vi "OdorSystem-V2.2.vi"() -> ()   [LabVIEW 2019]
doc: "Control odor delivery system in Setup B\n\nNeeds Labview 2019 and DAQmx 19! So that it is compatible with scanimage on Setup B\n\nBy Dr. Jan Eckhardt, Group Friedrich, FMI Basel"
uses:
  StatesEnum.ctl
  <vilib>/vision/Avi.llb/IMAQ AVI2 Refnum.ctl
  <vilib>/Utility/error.llb/DialogType.ctl
  <vilib>/DAQmx/write.llb/DAQmx Write (Digital 1D Bool NChan 1Samp 1Line).vi
  <vilib>/DAQmx/write.llb/DAQmx Write (Digital Wfm 1Chan NSamp).vi
  <vilib>/DAQmx/read.llb/DAQmx Read (Counter U32 1Chan 1Samp).vi
  <vilib>/DAQmx/read.llb/DAQmx Read (Digital 1D Bool 1Chan 1Samp).vi
  <vilib>/Utility/config.llb/Read Key (Double).vi
  <vilib>/Utility/config.llb/Read Key (I32).vi
  <vilib>/Utility/config.llb/Read Key (Boolean).vi
  <vilib>/Utility/config.llb/Read Key (String).vi
  <vilib>/DAQmx/miscellaneous.llb/DAQmx Fill In Error Info.vi
  <vilib>/DAQmx/create/channels.llb/DAQmx Create Channel (CO-Pulse Generation-Frequency).vi
  <vilib>/Waveform/DWDTOps.llb/Digital Pattern Generator (Single Value).vi
  <vilib>/Waveform/DWDTOps.llb/DWDT Append Digital Samples.vi
  <vilib>/DAQmx/configure/timing.llb/DAQmx Timing (Implicit).vi
  <vilib>/DAQmx/create/channels.llb/DAQmx Create Channel (CI-Count Edges).vi
  <vilib>/DAQmx/configure/timing.llb/DAQmx Timing (Sample Clock).vi
  <vilib>/Waveform/DWDTOps.llb/DWDT Append Digital Signals.vi
  <vilib>/Waveform/DWDTOps.llb/DWDT Digital to Boolean Array.vi
  <vilib>/DAQmx/create/channels.llb/DAQmx Create Channel (DO-Digital Output).vi
  <vilib>/Waveform/DWDTOps.llb/DWDT Uncompress Digital.vi
  <resource>/objmgr/daqmx.rc
  <vilib>/Utility/config.llb/NI_LVConfig.lvlib
  <vilib>/vision/driver/NI_Vision_Acquisition_Software.lvlib
panel:
  in  "Save Video as":enum32{"Bin", "Avi"}(radio)
  out "Experiment Refnum":T1
  in  "Start Recording":bool
  in  "Avi Codec":u16(ring)=3 items=["Intel IYUV codec", "Microsoft Video 1", "FF Video Codec 1 (FFV1) (NI Vision)", "Motion JPEG (NI Vision)", "VP8 (NI Vision)", "VP9 (NI Vision)", "Y800 Uncompressed Grey Scale (NI Vision)", "YUV 4:2:0 Planar (NI Vision)"]
  in  "Basename":string="Test5_Fish2_comparison"
  in  "Video path":path=path "C:/Users/eckhjan/Setup-C/output/JanVersion"
  in  "Image Type":T2 items=["Grayscale (U8)", "Grayscale (I16)", "Grayscale (SGL)", "Complex (CSG)", "RGB (U32)", "HSL (U32)", "RGB (U64)", "Grayscale (U16)"]
  out "Image":T3(plugin-control)
  in  "Time between frames (ms)":dbl(slide)=19.0 step=1.0 scale=0.0..100.0
  in  "Camera Name":refnum<k21> caption="IMAQdx Session"
  out "Loaded experiment":string
  in  "Load exp. ini":bool
  in  "Use Default valve":bool=TRUE
  in  "Selected default valve":u8(knob)=8 min=1 max=8 step=1 scale=1.0..8.0
  out "Framecount":u32
  in  "Image count filepath":path
  out "Experiment running":bool
  out "State":T4
  in  "Select experiment":enum32{"Single trial", "Trial series"}(tab)
  out "Time elapsed":dbl format="%.1f"
  in  "Start single trial":bool
  out "single trial done":bool
  in  "Select valve":u8(knob)=1 min=1 max=8 step=1 scale=1.0..8.0
  out "Pause elapsed time":dbl format="%#.1f"
  out "In between trials":bool
  out "Trial elapsed time":dbl format="%.1f"
  out "Total elapsed time":dbl format="%.1f"
  out "Estimated total time":dbl
  out "Current list index":i32
  out "Current Valve":u8
  in  "Time between trials":u16=10 min=1 max=900 step=1
  in  "Start trial series":bool
  in  "Valve order list":i8[](array[numeric]) min=1 max=8 step=1
  out "Digitaler output":digitalwaveform(graph)
  out "Stop Boolesch":bool
  in  "Total trial time":dbl=20.0 min=1.0 step=0.1
  in  "Valve opening time":dbl=10.0 min=0.0 step=0.1
  in  "Valve delay":dbl=2.0 min=0.0 step=0.1
  in  "Stopp":bool
  # "All times are in second!"
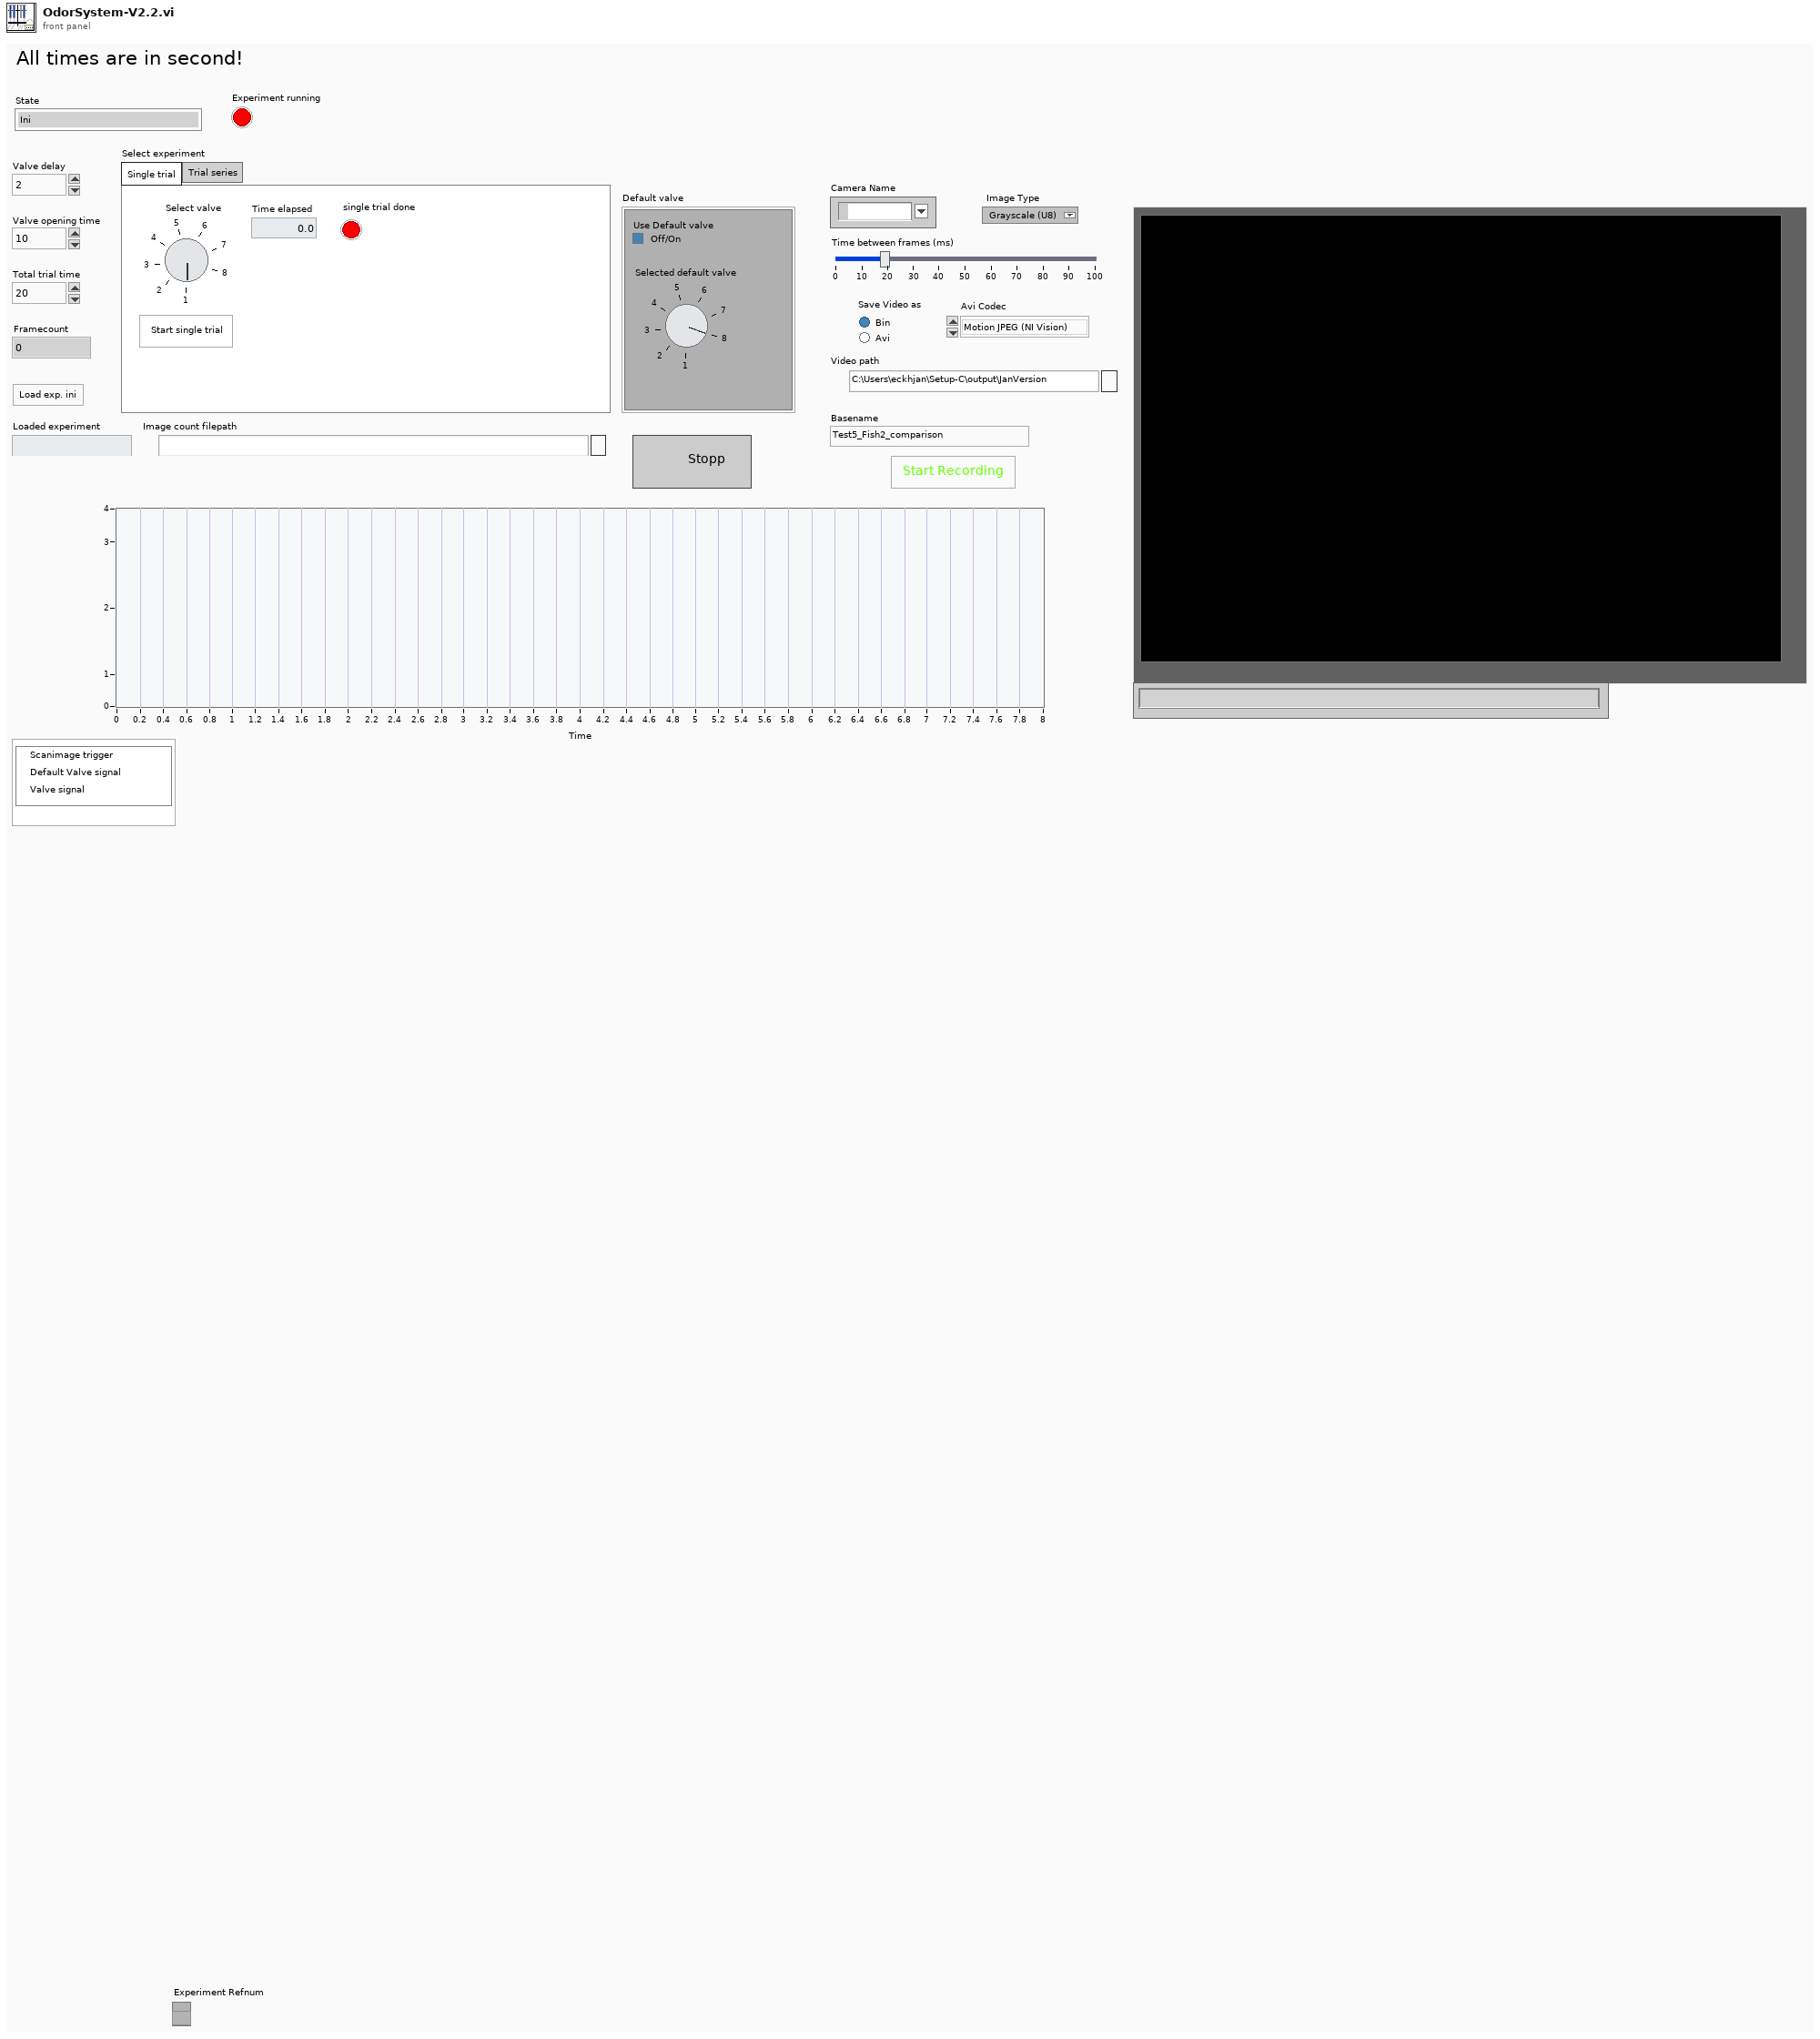
[diagram p1: front panel]
types:
  T1 = typedef "IMAQ AVI2 Refnum.ctl" = refnum<k20>
  T2 = typedef "Image Type" = u32
  T3 = typedef "IMAQ Image.ctl" = refnum<image>
  T4 = typedef "StatesEnum.ctl" = enum16{"Ini", "Standby", "Start Trial", "Start trial series", "Stop"}
  T5 = typedef "IMAQdx.ctl" = refnum<k21>
  T6 = enum8{"Enabled", "Disabled", "Disabled and Grayed Out"}
  T7 = enum32{"Page Enabled", "Page Disabled", "Page Disabled & Grayed"}
  T8 = enum16{"open", "replace", "create", "open or create", "replace or create", "replace or create with confirmation"}
  T9 = enum16{"big-endian, network order", "native, host order", "little-endian"}
  T10 = typedef "NI_LVConfig.lvlib/Config Data RefNum.ctl" = refnum<k1>
  T11 = typedef "DialogType.ctl" = u16
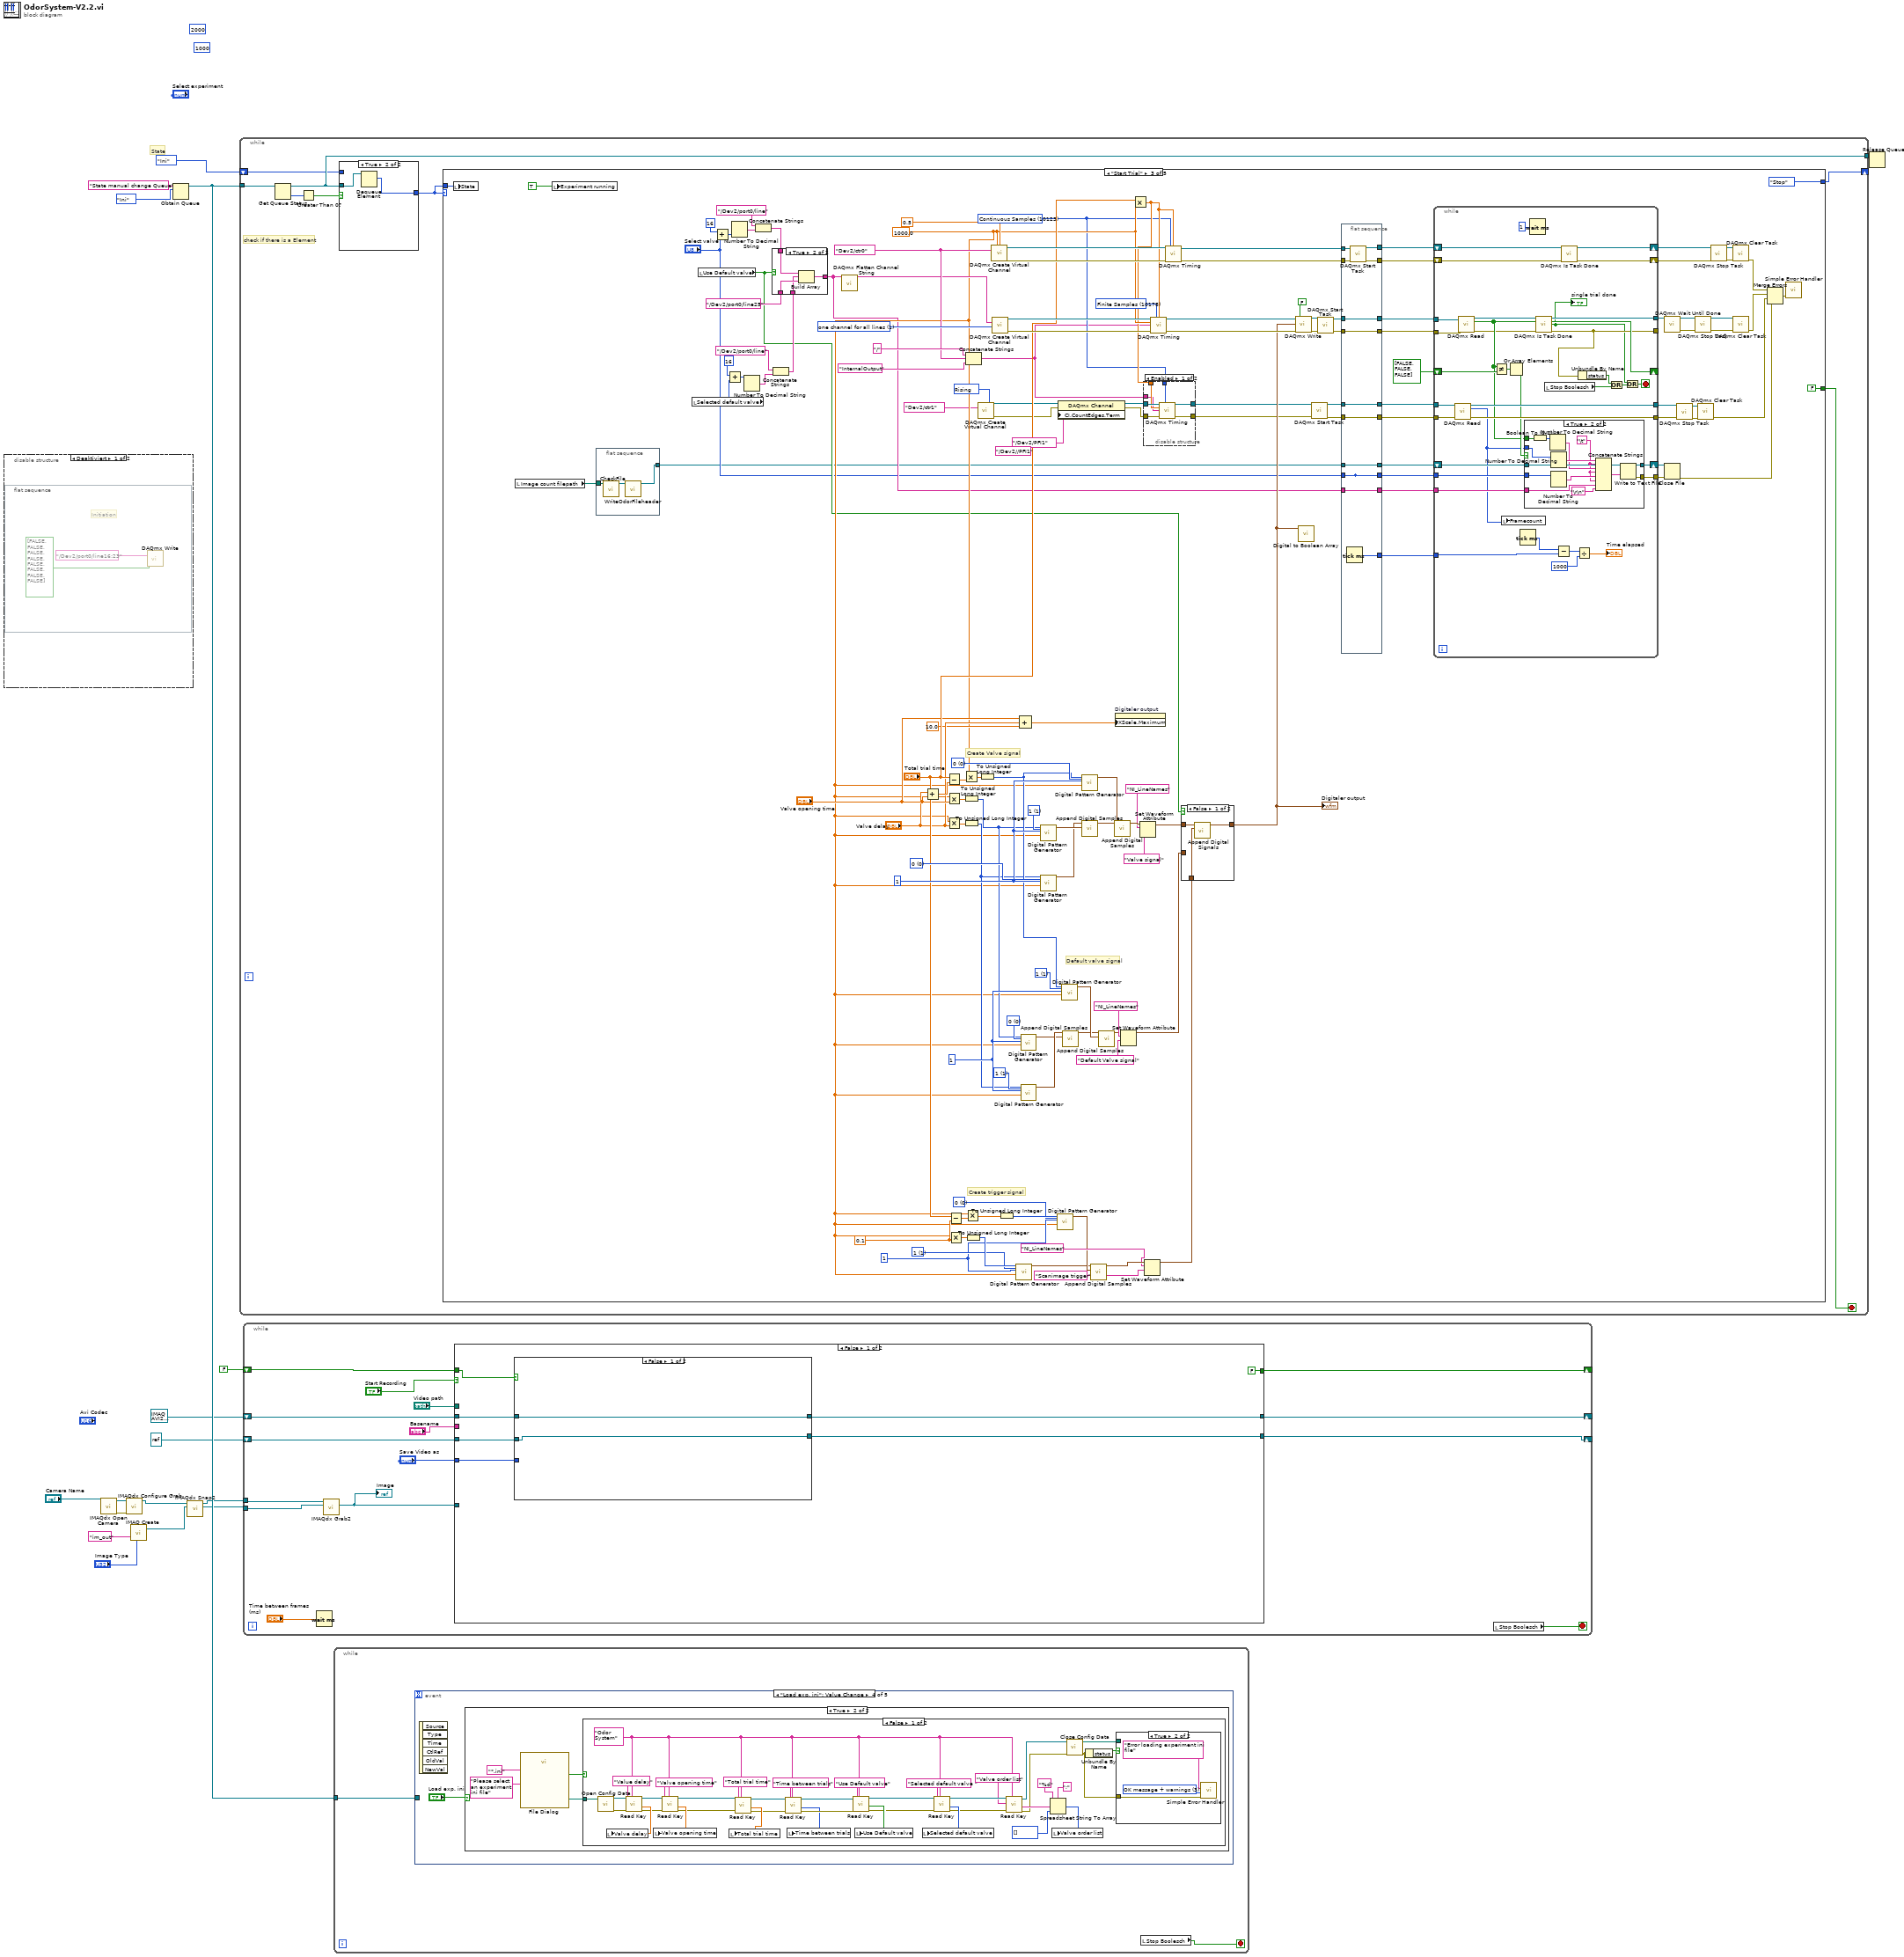
[diagram p0: block diagram]
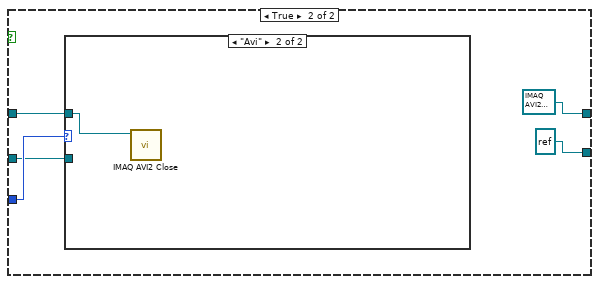
[diagram p2: hidden frame]
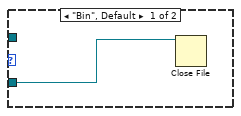
[diagram p3: hidden frame]
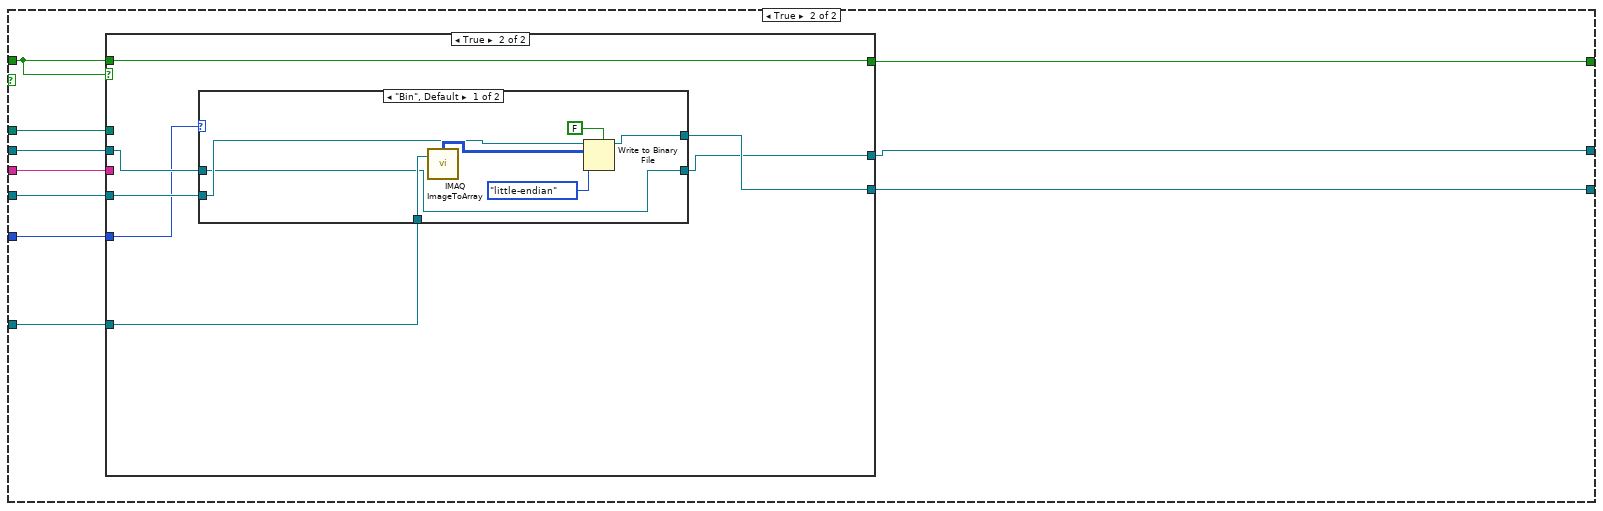
[diagram p4: hidden frame]
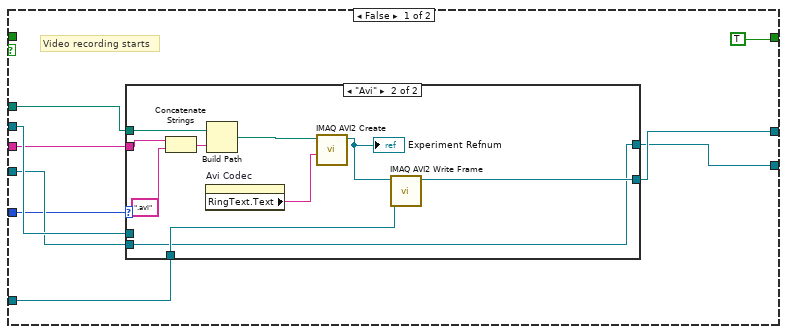
[diagram p5: hidden frame]
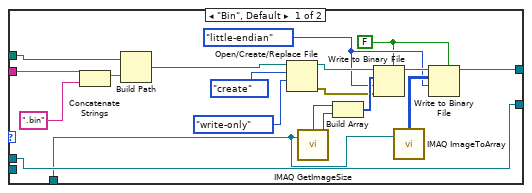
[diagram p6: hidden frame]
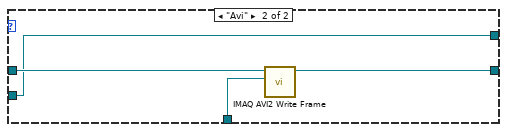
[diagram p7: hidden frame]
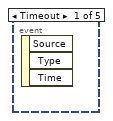
[diagram p9: hidden frame]
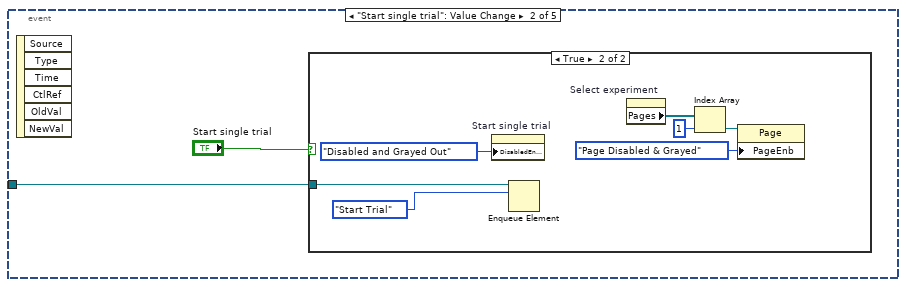
[diagram p10: hidden frame]
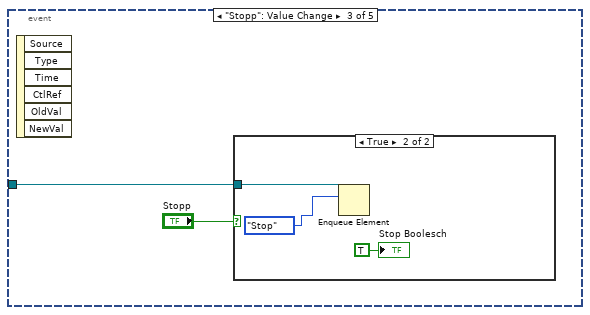
[diagram p12: hidden frame]
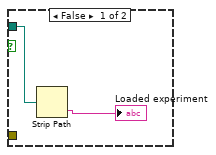
[diagram p15: hidden frame]
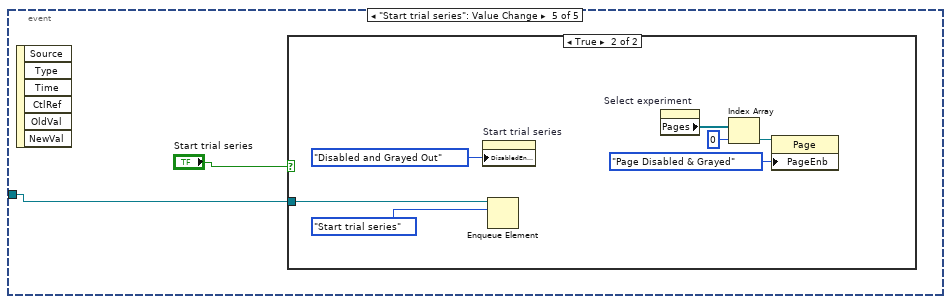
[diagram p17: hidden frame]
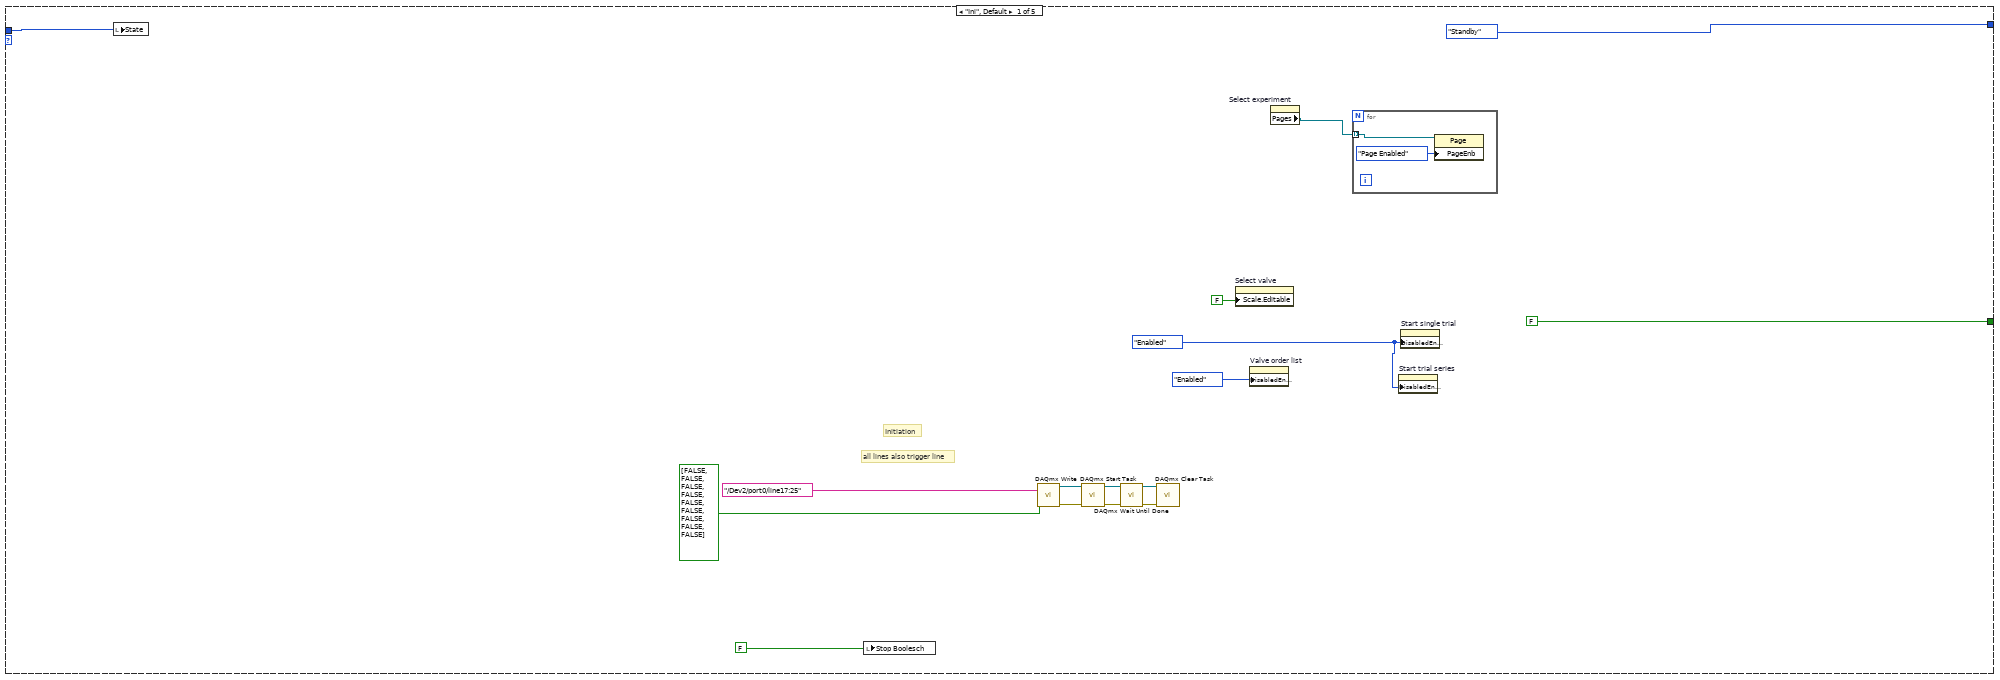
[diagram p20: hidden frame]
diagram:
  (unwired) u32 2000 ("number of samples")
  (unwired) u32 1000 ("number of samples")
  # "State"
  n1 = disable-structure shown="Deaktiviert" {
    frame Disabled {
      n2 = flat-sequence {
        frame #0 {
          # "Initiation"
          n3 = call-poly <vilib>:"DAQmx Write.vi"("task/channels in"="/Dev2/port0/line16:23" ("string"), "data"=bool[] [FALSE, FALSE, FALSE, FALSE, FALSE, FALSE, FALSE, FALSE]) -> ()  [unwired: 11 in, 3 out]
        }
      }
    }
    frame Enabled {
    }
  }
  n4 = call <vilib>:"IMAQdx Open Camera.vi"("Session In"="Camera Name") -> ("error out"=w11:errorcluster, "Session Out"=w12:T5)  [unwired: 9 in]
  n5 = call <vilib>:"IMAQdx Configure Grab.vi"("error in"=w11, "Session In"=w12) -> ("Session Out"=w5:T5)  [unwired: 8 in, 1 out]
  n6 = call "IMAQ Create"("Image Name"="im_out", "Image Type"="Image Type") -> ("New Image"=w4:T3)  [unwired: 3 in, 1 out]
  n7 = Obtain Queue(name (unnamed)="State manual change Queue", element data type=StatesEnum."Ini" ("Enum")) -> (queue out=w16:refnum<queue>)  [unwired: 3 in, 2 out]
  n8 = call <vilib>:"IMAQdx Snap2.vi"("Image In"=w4, "Session In"=w5) -> ("Image Out"=w2:T3, "Session Out"=w3:T5)  [unwired: 7 in, 1 out]
  n9 = while {
    tunnel: w16 -> [w25]
    tunnel: [w24] -> w15
    shift-right: [w20] -> _
    shift-left: StatesEnum."Ini" -> [w21]
    stop <- w23 stop-if-true
    # "check if there is a Element"
    n10 = Get Queue Status(queue=w25) -> (queue out=w24:refnum<queue>, # elements in queue=w27:i32)  [unwired: 2 in, 6 out]
    n11 = Greater Than 0?(x=w27) -> (x > 0?=w26:bool)
    n12 = case shown="True" w26 {
      tunnel: w24 -> [_ w30]
      tunnel: w21 -> [w28 _]
      tunnel: [w28 w29] -> w22
      frame False {
      }
      frame True {
        n13 = Dequeue Element(queue=w30) -> (element=w29:T4)  [unwired: 2 in, 3 out]
      }
    }
    n14 = case shown="\"Start Trial\"" w22 {
      tunnel: w22 -> [w41 w49 w127 w288 w607]
      tunnel: [FALSE ("Stop Boolesch") FALSE ("Stop Boolesch") FALSE ("Stop Boolesch") FALSE ("Stop Boolesch") w609] -> w23
      tunnel: [StatesEnum."Standby" ("Enum") w49 StatesEnum."Stop" ("Enum") StatesEnum."Stop" ("Enum") StatesEnum."Standby" ("Enum")] -> w20
      frame "Ini", Default {
        w34 = T6."Enabled" ("Deaktiviert")
        # "all lines also trigger line"
        # "Initiation"
        n15 = local write "State"(w41) -> ()
        n16 = local write "Stop Boolesch"(FALSE ("Stop Boolesch")) -> ()
        n17 = call-poly <vilib>:"DAQmx Write.vi"("task/channels in"="/Dev2/port0/line17:25" ("string"), "data"=bool[] [FALSE, FALSE, FALSE, FALSE, FALSE, FALSE, FALSE, FALSE, FALSE]) -> ("task out"=w36:refnum<k21>, "error out"=w35:errorcluster)  [unwired: 11 in, 1 out]
        n18 = call <vilib>:"DAQmx Start Task.vi"("task/channels in"=w36, "error in"=w35) -> ("task out"=w40:refnum<k21>, "error out"=w38:errorcluster)  [unwired: 12 in]
        n19 = call <vilib>:"DAQmx Wait Until Done.vi"("task/channels in"=w40, "error in"=w38) -> ("task out"=w39:refnum<k21>, "error out"=w37:errorcluster)  [unwired: 12 in]
        n20 = call <vilib>:"DAQmx Clear Task.vi"("task in"=w39, "error in"=w37) -> ()  [unwired: 13 in, 1 out]
        n21 = property on="Select valve" class="Knob (strict)"("Scale.Editable"=FALSE ("Skala.Editierbar")) -> ()  [unwired: 2 in, 2 out]
        n22 = property on="Valve order list" class="Arr (strict)"("DisabledEnum"=T6."Enabled" ("Deaktiviert")) -> ()  [unwired: 2 in, 2 out]
        n23 = property on="Select experiment" class="TabCtl (strict)"() -> ("Pages"=w32:refnum<vi>[])  [unwired: 2 in, 2 out]
        n24 = for {
          tunnel: w32 -> [w47] mode=indexing
          n25 = property class="Page"(reference=w47, "PageEnb"=T7."Page Enabled" ("Aktiv-Status der Seite")) -> ()  [unwired: 1 in, 2 out]
        }
        n26 = property on="Start trial series" class="Bool"("DisabledEnum"=w34) -> ()  [unwired: 2 in, 2 out]
        n27 = property on="Start single trial" class="Bool"("DisabledEnum"=w34) -> ()  [unwired: 2 in, 2 out]
      }
      frame "Standby" {
        n28 = local write "State"(w49) -> ()
        n29 = Wait (ms)(milliseconds to wait=u32 1 ("Zu wartende ms")) -> ()  [unwired: 1 out]
      }
      frame "Start Trial" {
        w95 = 10178 items=["Finite Samples"=10178, "Continuous Samples"=10123, "Hardware Timed Single Point"=12522] ("sample mode")
        (unwired) "/Dev2//PFI1" ("string")
        w105 = 10280 items=["Rising"=10280, "Falling"=10171] ("edge")
        w115 = u32 1 ("number of signals")
        w118 = u8 1 items=["0", "1", "Z", "L", "H", "X", "T", "V"] ("value")
        w117 = u8 0 items=["0", "1", "Z", "L", "H", "X", "T", "V"] ("value")
        w116 = u8 1 items=["0", "1", "Z", "L", "H", "X", "T", "V"] ("value")
        w147 = 0.1 ("y")
        w150 = u32 1 ("number of signals")
        w152 = u8 0 items=["0", "1", "Z", "L", "H", "X", "T", "V"] ("value")
        w151 = u8 1 items=["0", "1", "Z", "L", "H", "X", "T", "V"] ("value")
        w167 = tag "Dev2/ctr0" ("counter")
        w111 = 1000.0 ("frequency")
        w171 = u32 1 ("number of signals")
        w172 = u8 0 items=["0", "1", "Z", "L", "H", "X", "T", "V"] ("value")
        w173 = u8 1 items=["0", "1", "Z", "L", "H", "X", "T", "V"] ("value")
        w174 = u8 0 items=["0", "1", "Z", "L", "H", "X", "T", "V"] ("value")
        w185 = 1 items=["one channel for each line", "one channel for all lines"] ("line grouping")
        w96 = 10123 items=["Finite Samples"=10178, "Continuous Samples"=10123] ("sample mode")
        # "Default valve signal"
        # "Create trigger signal"
        # "Create Valve signal"
        n30 = local write "State"(w127) -> ()
        n31 = local read "Image count filepath"() -> (w66:path)
        n32 = local write "Experiment running"(TRUE ("Experiment running")) -> ()
        n33 = flat-sequence {
          tunnel: w66 -> [w194]
          tunnel: [w192] -> w67
          frame #0 {
            n34 = call "CheckFile.vi"("Image count filepath"=w194) -> ("Byte Stream File out"=w193:refnum<file>)  [unwired: 10 in]
            n35 = call "WriteOdorFileheader.vi"("Byte Stream File in"=w193) -> ("Byte Stream File out"=w192:refnum<file>)  [unwired: 10 in]
          }
        }
        n36 = local read "Selected default valve"() -> (w85:u8)
        n37 = local read "Use Default valve"() -> (w86:bool)
        n38 = Add(x=i8 16, y="Select valve") -> (x+y=w159:u8)
        n39 = Add(x=i8 16, y=w85) -> (x+y=w92:u8)
        n40 = Number To Decimal String(number=w159) -> (decimal integer string=w160:string)  [unwired: 1 in]
        n41 = Number To Decimal String(number=w92) -> (decimal integer string=w91:string)  [unwired: 1 in]
        n42 = Concatenate Strings("/Dev2/port0/line" ("string"), w160) -> (w89:string)
        n43 = Concatenate Strings("/Dev2/port0/line" ("string"), w91) -> (w87:string)
        n44 = case shown="True" w86 {
          tunnel: w89 -> [w248 w251]
          tunnel: "/Dev2/port0/line25" ("string") -> [w247 w250]
          tunnel: [w246 w252] -> w70
          tunnel: w87 -> [_ w249]
          frame False {
            n45 = Build Array(w248, w247) -> (w246:string[])
          }
          frame True {
            n46 = Build Array(w251, w249, w250) -> (w252:string[])
          }
        }
        n47 = call <vilib>:"DAQmx Flatten Channel String.vi"("names in"=w70) -> ("names out"=w149:string)  [unwired: 13 in, 1 out]
        n48 = Add(x="Valve delay", y="Valve opening time") -> (x+y=w163:dbl)
        n49 = Subtract(x="Total trial time", y=w163) -> (x-y=w162:dbl)
        n50 = Multiply(x=w111, y="Valve opening time") -> (x*y=w165:dbl)
        n51 = Multiply(x=w111, y="Valve delay") -> (x*y=w166:dbl)
        n52 = Subtract(x="Total trial time", y=w147) -> (x-y=w157:dbl)
        n53 = Multiply(x=w111, y=w147) -> (x*y=w153:dbl)
        n54 = Multiply(x=w111, y=w162) -> (x*y=w164:dbl)
        n55 = To Unsigned Long Integer(number=w165) -> (unsigned 32bit integer=w113:u32)
        n56 = To Unsigned Long Integer(number=w166) -> (unsigned 32bit integer=w112:u32)
        n57 = Multiply(x=w111, y=w157) -> (x*y=w155:dbl)
        n58 = To Unsigned Long Integer(number=w153) -> (unsigned 32bit integer=w154:u32)
        n59 = Concatenate Strings("/", w167, "InternalOutput" ("string")) -> (w94:string)
        n60 = call-poly <vilib>:"DAQmx Create Virtual Channel.vi"("edge"=w105, "counter"=tag "Dev2/ctr1") -> ("task out"=w103:refnum<k21>, "error out"=w100:errorcluster)  [unwired: 12 in]
        n61 = To Unsigned Long Integer(number=w164) -> (unsigned 32bit integer=w114:u32)
        n62 = call-poly <vilib>:"DAQmx Create Virtual Channel.vi"("frequency"=w111, "duty cycle"=0.5, "counter"=w167) -> ("task out"=w188:refnum<k21>, "error out"=w189:errorcluster)  [unwired: 11 in]
        n63 = call-poly <vilib>:"DAQmx Create Virtual Channel.vi"("lines"=w149, "line grouping"=w185) -> ("task out"=w191:refnum<k21>, "error out"=w190:errorcluster)  [unwired: 12 in]
        n64 = To Unsigned Long Integer(number=w155) -> (unsigned 32bit integer=w156:u32)
        n65 = call-poly <vilib>:"Digital Pattern Generator.vi"("value"=w151, "sample rate"=w111, "number of signals"=w150, "number of samples"=w154) -> ("digital waveform"=w135:digitalwaveform)  [unwired: 6 in, 1 out]
        n66 = Compound Arithmetic op=ADD("Valve opening time", "Valve delay", 10.0 ("Wert")) -> (w128:dbl)
        n67 = call-poly <vilib>:"Digital Pattern Generator.vi"("value"=w117, "sample rate"=w111, "number of signals"=w115, "number of samples"=w113) -> ("digital waveform"=w122:digitalwaveform)  [unwired: 6 in, 1 out]
        n68 = call-poly <vilib>:"Digital Pattern Generator.vi"("value"=w116, "sample rate"=w111, "number of signals"=w115, "number of samples"=w112) -> ("digital waveform"=w123:digitalwaveform)  [unwired: 6 in, 1 out]
        n69 = call-poly <vilib>:"Digital Pattern Generator.vi"("value"=w173, "sample rate"=w111, "number of signals"=w171, "number of samples"=w113) -> ("digital waveform"=w140:digitalwaveform)  [unwired: 6 in, 1 out]
        n70 = call-poly <vilib>:"Digital Pattern Generator.vi"("value"=w174, "sample rate"=w111, "number of signals"=w171, "number of samples"=w112) -> ("digital waveform"=w139:digitalwaveform)  [unwired: 6 in, 1 out]
        n71 = call-poly <vilib>:"Digital Pattern Generator.vi"("value"=w152, "sample rate"=w111, "number of signals"=w150, "number of samples"=w156) -> ("digital waveform"=w136:digitalwaveform)  [unwired: 6 in, 1 out]
        n72 = property class="DAQmx Channel"(reference=w103, error in=w100, "CI.CountEdges.Term"=tag "/Dev2/PFI1") -> (reference out=w102:refnum<k21>, error out=w101:errorcluster)
        n73 = call-poly <vilib>:"Digital Pattern Generator.vi"("value"=w118, "sample rate"=w111, "number of signals"=w115, "number of samples"=w114) -> ("digital waveform"=w125:digitalwaveform)  [unwired: 6 in, 1 out]
        n74 = call-poly <vilib>:"Append Digital Samples.vi"("digital waveform B"=w122, "digital waveform A"=w123) -> ("digital waveform out"=w124:digitalwaveform)  [unwired: 8 in, 1 out]
        n75 = call-poly <vilib>:"Digital Pattern Generator.vi"("value"=w172, "sample rate"=w111, "number of signals"=w171, "number of samples"=w114) -> ("digital waveform"=w137:digitalwaveform)  [unwired: 6 in, 1 out]
        n76 = call-poly <vilib>:"Append Digital Samples.vi"("digital waveform B"=w140, "digital waveform A"=w139) -> ("digital waveform out"=w138:digitalwaveform)  [unwired: 8 in, 1 out]
        n77 = call-poly <vilib>:"Append Digital Samples.vi"("digital waveform B"=w136, "digital waveform A"=w135) -> ("digital waveform out"=w146:digitalwaveform)  [unwired: 8 in, 1 out]
        n78 = call-poly <vilib>:"Append Digital Samples.vi"("digital waveform B"=w125, "digital waveform A"=w124) -> ("digital waveform out"=w119:digitalwaveform)  [unwired: 8 in, 1 out]
        n79 = call-poly <vilib>:"Append Digital Samples.vi"("digital waveform B"=w137, "digital waveform A"=w138) -> ("digital waveform out"=w143:digitalwaveform)  [unwired: 8 in, 1 out]
        n80 = property on="Digitaler output" class="DigitalGraph (strict)"("XScale.Maximum"=w128) -> ()  [unwired: 2 in, 2 out]
        n81 = Set Waveform Attribute(5:"Default Valve signal", 6:"NI_LineNames" ("name"), 7:w119) -> (3:w107:digitalwaveform)  [unwired: 1 in, 2 out]
        n82 = Multiply(x="Total trial time", y=w111) -> (x*y=w97:dbl)
        n83 = Set Waveform Attribute(5:"Valve signal", 6:"NI_LineNames" ("name"), 7:w143) -> (3:w110:digitalwaveform)  [unwired: 1 in, 2 out]
        n84 = disable-structure shown="Enabled" {
          disable-tunnel: w102 -> [w259 w261]
          disable-tunnel: w97 -> [w258 _]
          disable-tunnel: w94 -> [w257 _]
          disable-tunnel: w101 -> [w256 w260]
          disable-tunnel: [w255 w261] -> w104
          disable-tunnel: [w254 w260] -> w98
          disable-tunnel: w96 -> [w253 _]
          frame Enabled {
            n85 = call-poly <vilib>:"DAQmx Timing.vi"("task/channels in"=w259, "sample mode"=w253, "rate"=w258, "source"=w257, "error in"=w256) -> ("task out"=w255:refnum<k21>, "error out"=w254:errorcluster)  [unwired: 9 in]
          }
          frame Disabled {
          }
        }
        n86 = Set Waveform Attribute(5:"Scanimage trigger", 6:"NI_LineNames" ("name"), 7:w146) -> (3:w108:digitalwaveform)  [unwired: 1 in, 2 out]
        n87 = call-poly <vilib>:"DAQmx Timing.vi"("task/channels in"=w191, "sample mode"=w95, "samples per channel"=w97, "rate"=w111, "source"=w94, "error in"=w190) -> ("task out"=w182:refnum<k21>, "error out"=w181:errorcluster)  [unwired: 8 in]
        n88 = call-poly <vilib>:"DAQmx Timing.vi"("task/channels in"=w188, "sample mode"=w96, "samples per channel"=w97, "error in"=w189) -> ("task out"=w186:refnum<k21>, "error out"=w187:errorcluster)  [unwired: 10 in]
        n89 = case shown="False" w86 {
          tunnel: w110 -> [w264 w269]
          tunnel: w108 -> [w263 w267]
          tunnel: [w262 w268] -> w109
          tunnel: w107 -> [_ w266]
          frame False {
            n90 = call-poly <vilib>:"Append Digital Signals.vi"("digital waveform (low bits)"=w263, "digital waveform (high bits)"=w264) -> ("digital waveform out"=w262:digitalwaveform)  [unwired: 8 in, 1 out]
          }
          frame True {
            n91 = call-poly <vilib>:"Append Digital Signals.vi"("digital waveform (low bits)"=w267, "digital waveform (high bits)"=w266) -> ("digital waveform out"=w265:digitalwaveform)  [unwired: 8 in, 1 out]
            n92 = call-poly <vilib>:"Append Digital Signals.vi"("digital waveform (low bits)"=w265, "digital waveform (high bits)"=w269) -> ("digital waveform out"=w268:digitalwaveform)  [unwired: 8 in, 1 out]
          }
        }
        "Digitaler output" <- w109
        n93 = call-poly <vilib>:"DAQmx Write.vi"("task/channels in"=w182, "auto start"=FALSE, "data"=w109, "error in"=w181) -> ("task out"=w180:refnum<k21>, "error out"=w179:errorcluster)  [unwired: 9 in, 1 out]
        n94 = call-poly <vilib>:"Digital to Boolean Array.vi"("digital waveform"=w109) -> ()  [unwired: 9 in, 2 out]
        n95 = call <vilib>:"DAQmx Start Task.vi"("task/channels in"=w104, "error in"=w98) -> ("task out"=w78:refnum<k21>, "error out"=w77:errorcluster)  [unwired: 12 in]
        n96 = call <vilib>:"DAQmx Start Task.vi"("task/channels in"=w180, "error in"=w179) -> ("task out"=w184:refnum<k21>, "error out"=w183:errorcluster)  [unwired: 12 in]
        n97 = flat-sequence {
          tunnel: [w281] -> w84
          tunnel: [w280] -> w83
          tunnel: w187 -> [w279]
          tunnel: w186 -> [w278]
          tunnel: [w277] -> w82
          tunnel: w184 -> [w277]
          tunnel: [w276] -> w81
          tunnel: w183 -> [w276]
          tunnel: [w275] -> w74
          tunnel: [w274] -> w76
          tunnel: w78 -> [w274]
          tunnel: [w273] -> w75
          tunnel: w77 -> [w273]
          tunnel: [w272] -> w73
          tunnel: w70 -> [w272]
          tunnel: [w270] -> w72
          tunnel: [w270] -> _
          tunnel: [w271] -> w71
          tunnel: w67 -> [w271]
          tunnel: "Select valve" -> [w270]
          frame #0 {
            n98 = Tick Count (ms)() -> (millisecond timer value=w275:u32)
            n99 = call <vilib>:"DAQmx Start Task.vi"("task/channels in"=w278, "error in"=w279) -> ("task out"=w281:refnum<k21>, "error out"=w280:errorcluster)  [unwired: 12 in]
          }
        }
        n100 = while {
          shift-right: [w226] -> w80
          shift-left: w84 -> [w228]
          shift-right: [w225] -> w54
          shift-left: w83 -> [w227]
          tunnel: w82 -> [w224]
          tunnel: w81 -> [w215]
          tunnel: [w201] -> w79
          tunnel: [w199] -> _
          tunnel: w74 -> [w220]
          tunnel: w76 -> [w214]
          tunnel: w75 -> [w212]
          tunnel: [w213] -> w62
          tunnel: [w211] -> w61
          shift-right: [w207] -> _
          shift-left: bool[] [FALSE, FALSE, FALSE] ("data") -> [w210]
          shift-right: [w205] -> w65
          shift-left: w71 -> [w206]
          tunnel: w73 -> [w204]
          tunnel: w72 -> [w203]
          tunnel: [w202] -> w64
          stop <- w221 stop-if-true
          n101 = call-poly <vilib>:"DAQmx Read.vi"("task/channels in"=w214, "error in"=w212) -> ("task out"=w213:refnum<k21>, "data"=w195:u32, "error out"=w211:errorcluster)  [unwired: 11 in]
          n102 = call-poly <vilib>:"DAQmx Read.vi"("task/channels in"=w224, "error in"=w215) -> ("task out"=w216:refnum<k21>, "data"=w207:bool[], "error out"=w200:errorcluster)  [unwired: 11 in]
          n103 = Not Equal?(x=w207, y=w210) -> (x != y?=w209:bool[])
          n104 = local write "Framecount"(w195) -> ()
          n105 = Or Array Elements(Boolean array=w209) -> (logical OR=w208:bool)
          n106 = Tick Count (ms)() -> (millisecond timer value=w219:u32)
          n107 = case shown="True" w208 {
            tunnel: w207 -> [_ w242]
            tunnel: w195 -> [_ w240]
            tunnel: w206 -> [w231 w244]
            tunnel: [w231 w243] -> w205
            tunnel: w204 -> [_ w234]
            tunnel: w203 -> [_ w237]
            tunnel: [errorcluster {"status"=FALSE, "code"=0, "source"=""} ("error out") w233] -> w202
            frame False {
            }
            frame True {
              w235 = "\t"
              n108 = Boolean To (0,1)(Boolean=w242) -> (0, 1=w241:i16[])
              n109 = Number To Decimal String(number=w241) -> (decimal integer string=w238:string[])  [unwired: 1 in]
              n110 = Number To Decimal String(number=w240) -> (decimal integer string=w239:string)  [unwired: 1 in]
              n111 = Number To Decimal String(number=w237) -> (decimal integer string=w236:string)  [unwired: 1 in]
              n112 = Concatenate Strings(w239, w235, w238, w235, w236, w235, w234, "\r\n") -> (w245:string)
              n113 = Write to Text File(file (use dialog)=w244, text=w245) -> (refnum out=w243:refnum<file>, error out=w233:errorcluster)  [unwired: 2 in, 1 out]
            }
          }
          n114 = Wait (ms)(milliseconds to wait=u32 1 ("Zu wartende ms")) -> ()  [unwired: 1 out]
          n115 = call <vilib>:"DAQmx Is Task Done.vi"("task/channels in"=w216, "error in"=w200) -> ("task out"=w201:refnum<k21>, "task done?"=w197:bool, "error out"=w199:errorcluster)  [unwired: 11 in]
          "single trial done" <- w197
          n116 = local read "Stop Boolesch"() -> (w198:bool)
          n117 = Subtract(x=w219, y=w220) -> (x-y=w218:u32)
          n118 = call <vilib>:"DAQmx Is Task Done.vi"("task/channels in"=w228, "error in"=w227) -> ("task out"=w226:refnum<k21>, "error out"=w225:errorcluster)  [unwired: 11 in, 1 out]
          n119 = Divide(x=w218, y=u32 1000 ("x")) -> (x/y=→"Time elapsed":dbl)
          n120 = Unbundle By Name(w199) -> ("status"=w222:bool)
          n121 = Or(x=w222, y=w198) -> (x .or. y?=w229:bool)
          n122 = Or(x=w197, y=w229) -> (x .or. y?=w221:bool)
        }
        n123 = call <vilib>:"DAQmx Wait Until Done.vi"("task/channels in"=w79) -> ("task out"=w131:refnum<k21>, "error out"=w57:errorcluster)  [unwired: 13 in]
        n124 = Close File(refnum=w65, error in=w64) -> (error out=w52:errorcluster)  [unwired: 1 out]
        n125 = call <vilib>:"DAQmx Stop Task.vi"("task/channels in"=w62, "error in"=w61) -> ("task out"=w63:refnum<k21>, "error out"=w60:errorcluster)  [unwired: 12 in]
        n126 = call <vilib>:"DAQmx Stop Task.vi"("task/channels in"=w131, "error in"=w57) -> ("task out"=w58:refnum<k21>, "error out"=w56:errorcluster)  [unwired: 12 in]
        n127 = call <vilib>:"DAQmx Clear Task.vi"("task in"=w63, "error in"=w60) -> ("error out"=w59:errorcluster)  [unwired: 13 in]
        n128 = call <vilib>:"DAQmx Stop Task.vi"("task/channels in"=w80, "error in"=w54) -> ("task out"=w55:refnum<k21>, "error out"=w53:errorcluster)  [unwired: 12 in]
        n129 = call <vilib>:"DAQmx Clear Task.vi"("task in"=w55, "error in"=w53) -> ("error out"=w177:errorcluster)  [unwired: 13 in]
        n130 = call <vilib>:"DAQmx Clear Task.vi"("task in"=w58, "error in"=w56) -> ("error out"=w176:errorcluster)  [unwired: 13 in]
        n131 = Merge Errors(w177, w176, w59, w52) -> (w175:errorcluster)
        n132 = call <vilib>:"Simple Error Handler.vi"("error in (no error)"=w175) -> ()  [unwired: 4 in, 5 out]
      }
      frame "Start trial series" {
        w284 = T6."Disabled" ("Deaktiviert")
        n133 = property on="Valve order list" class="Arr (strict)"("DisabledEnum"=w284) -> ()  [unwired: 2 in, 2 out]
        n134 = property on="Image count filepath" class="Path"("DisabledEnum"=w284) -> ()  [unwired: 2 in, 2 out]
        n135 = for {
          tunnel: "Valve order list" -> [w365] mode=indexing
          shift-right: [w361] -> _
          shift-left: _ -> [w363]
          tunnel: "Image count filepath" -> [w346]
          shift-right: [w345] -> w283
          shift-left: _ -> [w344]
          tunnel: [w343] -> w282
          i -> [w370]
          stop <- w374 stop-if-true
          w301 = 10178 items=["Finite Samples"=10178, "Continuous Samples"=10123, "Hardware Timed Single Point"=12522] ("sample mode")
          w328 = u32 1 ("number of signals")
          w331 = u8 1 items=["0", "1", "Z", "L", "H", "X", "T", "V"] ("value")
          w330 = u8 0 items=["0", "1", "Z", "L", "H", "X", "T", "V"] ("value")
          w329 = u8 1 items=["0", "1", "Z", "L", "H", "X", "T", "V"] ("value")
          (unwired) "/Dev2//PFI1" ("string")
          w358 = 10280 items=["Rising"=10280, "Falling"=10171] ("edge")
          w391 = 0.2 ("y")
          w393 = u32 1 ("number of signals")
          w395 = u8 0 items=["0", "1", "Z", "L", "H", "X", "T", "V"] ("value")
          w394 = u8 1 items=["0", "1", "Z", "L", "H", "X", "T", "V"] ("value")
          w410 = tag "Dev2/ctr0" ("counter")
          w327 = 1000.0 ("frequency")
          w417 = u32 1 ("number of signals")
          w294 = u8 1 items=["0", "1", "Z", "L", "H", "X", "T", "V"] ("value")
          w418 = u8 1 items=["0", "1", "Z", "L", "H", "X", "T", "V"] ("value")
          w293 = u8 0 items=["0", "1", "Z", "L", "H", "X", "T", "V"] ("value")
          w426 = 1 items=["one channel for each line", "one channel for all lines"] ("line grouping")
          w305 = 10123 items=["Finite Samples"=10178, "Continuous Samples"=10123] ("sample mode")
          # "Default valve signal"
          # "Create trigger signal"
          # "Create Valve signal"
          n136 = Equal?(x=0, y=w370) -> (x = y?=w364:bool)
          n137 = flat-sequence {
            tunnel: [w473] -> w298
            tunnel: w365 -> [w473]
            tunnel: w364 -> [w472]
            tunnel: w363 -> [w471]
            tunnel: w362 -> [w470]
            tunnel: [w469] -> w361
            tunnel: [w466] -> w351
            tunnel: w346 -> [w465]
            tunnel: w344 -> [w464]
            frame #0 {
              n138 = case shown="True" w472 {
                tunnel: [w475 w476] -> w469
                tunnel: w471 -> [w475 _]
                tunnel: w470 -> [_ w485]
                tunnel: w465 -> [_ w479]
                tunnel: [w474 w478] -> w466
                tunnel: w464 -> [w474 _]
                frame False {
                }
                frame True {
                  n139 = property on="Valve order list" class="Arr (strict)"() -> ("Value"=w483:i8[])  [unwired: 2 in, 2 out]
                  n140 = flat-sequence {
                    tunnel: w479 -> [w488]
                    tunnel: [w486] -> w477
                    tunnel: [w490] -> w478
                    tunnel: w477 -> [w490]
                    tunnel: [w489] -> w476
                    frame #0 {
                      n141 = call "CheckFile.vi"("Image count filepath"=w488) -> ("Byte Stream File out"=w487:refnum<file>)  [unwired: 10 in]
                      n142 = call "WriteOdorFileheader.vi"("Byte Stream File in"=w487) -> ("Byte Stream File out"=w486:refnum<file>)  [unwired: 10 in]
                    }
                    frame #1 {
                      n143 = Tick Count (ms)() -> (millisecond timer value=w489:u32)
                    }
                  }
                  n144 = local read "Time between trials"() -> (w480:u16)
                  n145 = Array Size(array=w483) -> (size(s)=w482:i32)
                  n146 = Add(x=w480, y=w485) -> (x+y=w481:dbl)
                  n147 = Multiply(x=w481, y=w482) -> (x*y=→"Estimated total time":dbl)
                }
              }
              n148 = local write "Pause elapsed time"(0.0 ("Pause elapsed time")) -> ()
              n149 = local write "In between trials"(FALSE ("In between trials")) -> ()
            }
          }
          n150 = local read "Total trial time"() -> (w362:dbl)
          n151 = Add(x=i8 16, y=w298) -> (x+y=w402:i8)
          n152 = Equal?(x=w298, y="Selected default valve") -> (x = y?=w291:bool)
          n153 = Number To Decimal String(number=w402) -> (decimal integer string=w403:string)  [unwired: 1 in]
          n154 = Select(t=10 ("f"), s=w291, f="Selected default valve") -> (s? t:f=w295:i32)
          n155 = Concatenate Strings("/Dev2/port0/line" ("string"), w403) -> (w319:string)
          n156 = Add(x=i8 16, y=w295) -> (x+y=w316:i32)
          n157 = Number To Decimal String(number=w316) -> (decimal integer string=w315:string)  [unwired: 1 in]
          n158 = Select(t=w294, s=w291, f=w293) -> (s? t:f=w292:u8)
          n159 = Concatenate Strings("/Dev2/port0/line" ("string"), w315) -> (w313:string)
          n160 = case shown="True" "Use Default valve" {
            tunnel: w319 -> [w436 w439]
            tunnel: "/Dev2/port0/line25" ("string") -> [w435 w438]
            tunnel: [w434 w440] -> w317
            tunnel: w313 -> [_ w437]
            frame False {
              n161 = Build Array(w436, w435) -> (w434:string[])
            }
            frame True {
              n162 = Build Array(w439, w437, w438) -> (w440:string[])
            }
          }
          n163 = local read "Valve opening time"() -> (w376:dbl)
          n164 = local read "Valve delay"() -> (w375:dbl)
          n165 = call <vilib>:"DAQmx Flatten Channel String.vi"("names in"=w317) -> ("names out"=w392:string, "error out"=w360:errorcluster)  [unwired: 13 in]
          n166 = call-poly <vilib>:"DAQmx Create Virtual Channel.vi"("edge"=w358, "counter"=tag "Dev2/ctr1") -> ("task out"=w342:refnum<k21>, "error out"=w339:errorcluster)  [unwired: 12 in]
          n167 = Add(x=w375, y=w376) -> (x+y=w406:dbl)
          n168 = call-poly <vilib>:"DAQmx Create Virtual Channel.vi"("frequency"=w327, "duty cycle"=0.5, "counter"=w410) -> ("task out"=w429:refnum<k21>, "error out"=w308:errorcluster)  [unwired: 11 in]
          n169 = call-poly <vilib>:"DAQmx Create Virtual Channel.vi"("lines"=w392, "line grouping"=w426, "error in"=w360) -> ("task out"=w433:refnum<k21>, "error out"=w432:errorcluster)  [unwired: 11 in]
          n170 = Concatenate Strings("/", w410, "InternalOutput" ("string")) -> (w357:string)
          n171 = Subtract(x=w362, y=w406) -> (x-y=w405:dbl)
          n172 = Multiply(x=w327, y=w376) -> (x*y=w408:dbl)
          n173 = Multiply(x=w327, y=w375) -> (x*y=w409:dbl)
          n174 = Subtract(x=w362, y=w391) -> (x-y=w400:dbl)
          n175 = Multiply(x=w327, y=w391) -> (x*y=w396:dbl)
          n176 = To Unsigned Long Integer(number=w409) -> (unsigned 32bit integer=w324:u32)
          n177 = Multiply(x=w327, y=w405) -> (x*y=w407:dbl)
          n178 = To Unsigned Long Integer(number=w408) -> (unsigned 32bit integer=w325:u32)
          n179 = Multiply(x=w327, y=w400) -> (x*y=w398:dbl)
          n180 = To Unsigned Long Integer(number=w396) -> (unsigned 32bit integer=w397:u32)
          n181 = To Unsigned Long Integer(number=w407) -> (unsigned 32bit integer=w326:u32)
          n182 = property class="DAQmx Channel"(reference=w342, error in=w339, "CI.CountEdges.Term"=tag "/Dev2/PFI1") -> (reference out=w341:refnum<k21>, error out=w340:errorcluster)
          n183 = To Unsigned Long Integer(number=w398) -> (unsigned 32bit integer=w399:u32)
          n184 = property class="DAQmx Channel"(reference=w429, error in=w308, "CO.Pulse.Term"=tag "/Dev2/PFI12") -> (reference out=w309:refnum<k21>, error out=w307:errorcluster)
          n185 = call-poly <vilib>:"Digital Pattern Generator.vi"("value"=w394, "sample rate"=w327, "number of signals"=w393, "number of samples"=w397) -> ("digital waveform"=w379:digitalwaveform)  [unwired: 6 in, 1 out]
          n186 = call-poly <vilib>:"Digital Pattern Generator.vi"("value"=w330, "sample rate"=w327, "number of signals"=w328, "number of samples"=w325) -> ("digital waveform"=w335:digitalwaveform)  [unwired: 6 in, 1 out]
          n187 = call-poly <vilib>:"Digital Pattern Generator.vi"("value"=w329, "sample rate"=w327, "number of signals"=w328, "number of samples"=w324) -> ("digital waveform"=w336:digitalwaveform)  [unwired: 6 in, 1 out]
          n188 = call-poly <vilib>:"Digital Pattern Generator.vi"("value"=w418, "sample rate"=w327, "number of signals"=w417, "number of samples"=w325) -> ("digital waveform"=w384:digitalwaveform)  [unwired: 6 in, 1 out]
          n189 = call-poly <vilib>:"Digital Pattern Generator.vi"("value"=w292, "sample rate"=w327, "number of signals"=w417, "number of samples"=w324) -> ("digital waveform"=w383:digitalwaveform)  [unwired: 6 in, 1 out]
          n190 = Compound Arithmetic op=ADD(w376, w375, 10.0 ("Wert")) -> (w377:dbl)
          n191 = property on="Digitaler output" class="DigitalGraph (strict)"("XScale.Maximum"=w377) -> ()  [unwired: 2 in, 2 out]
          n192 = call-poly <vilib>:"Digital Pattern Generator.vi"("value"=w395, "sample rate"=w327, "number of signals"=w393, "number of samples"=w399) -> ("digital waveform"=w380:digitalwaveform)  [unwired: 6 in, 1 out]
          n193 = call-poly <vilib>:"Digital Pattern Generator.vi"("value"=w331, "sample rate"=w327, "number of signals"=w328, "number of samples"=w326) -> ("digital waveform"=w338:digitalwaveform)  [unwired: 6 in, 1 out]
          n194 = call-poly <vilib>:"Append Digital Samples.vi"("digital waveform B"=w335, "digital waveform A"=w336) -> ("digital waveform out"=w337:digitalwaveform)  [unwired: 8 in, 1 out]
          n195 = call-poly <vilib>:"Digital Pattern Generator.vi"("value"=w292, "sample rate"=w327, "number of signals"=w417, "number of samples"=w326) -> ("digital waveform"=w381:digitalwaveform)  [unwired: 6 in, 1 out]
          n196 = call-poly <vilib>:"Append Digital Samples.vi"("digital waveform B"=w384, "digital waveform A"=w383) -> ("digital waveform out"=w382:digitalwaveform)  [unwired: 8 in, 1 out]
          n197 = disable-structure shown="Enabled" {
            disable-tunnel: w341 -> [w455 w457]
            disable-tunnel: w327 -> [w454 _]
            disable-tunnel: w357 -> [w453 _]
            disable-tunnel: w340 -> [w452 w456]
            disable-tunnel: [w451 w457] -> w356
            disable-tunnel: [w450 w456] -> w303
            disable-tunnel: w305 -> [w449 _]
            frame Enabled {
              n198 = call-poly <vilib>:"DAQmx Timing.vi"("task/channels in"=w455, "sample mode"=w449, "rate"=w454, "source"=w453, "error in"=w452) -> ("task out"=w451:refnum<k21>, "error out"=w450:errorcluster)  [unwired: 9 in]
            }
            frame Disabled {
            }
          }
          n199 = Multiply(x=w362, y=w327) -> (x*y=w300:dbl)
          n200 = call-poly <vilib>:"Append Digital Samples.vi"("digital waveform B"=w380, "digital waveform A"=w379) -> ("digital waveform out"=w390:digitalwaveform)  [unwired: 8 in, 1 out]
          n201 = call-poly <vilib>:"DAQmx Timing.vi"("task/channels in"=w433, "sample mode"=w301, "samples per channel"=w300, "rate"=w327, "source"=w357, "error in"=w432) -> ("task out"=w423:refnum<k21>, "error out"=w422:errorcluster)  [unwired: 8 in]
          n202 = call-poly <vilib>:"Append Digital Samples.vi"("digital waveform B"=w338, "digital waveform A"=w337) -> ("digital waveform out"=w332:digitalwaveform)  [unwired: 8 in, 1 out]
          n203 = call-poly <vilib>:"Append Digital Samples.vi"("digital waveform B"=w381, "digital waveform A"=w382) -> ("digital waveform out"=w387:digitalwaveform)  [unwired: 8 in, 1 out]
          n204 = call-poly <vilib>:"DAQmx Timing.vi"("task/channels in"=w309, "sample mode"=w305, "error in"=w307) -> ("task out"=w427:refnum<k21>, "error out"=w428:errorcluster)  [unwired: 11 in]
          n205 = Set Waveform Attribute(5:"Scanimage trigger", 6:"NI_LineNames" ("name"), 7:w390) -> (3:w321:digitalwaveform)  [unwired: 1 in, 2 out]
          n206 = Set Waveform Attribute(5:"Default Valve signal", 6:"NI_LineNames" ("name"), 7:w332) -> (3:w320:digitalwaveform)  [unwired: 1 in, 2 out]
          n207 = Set Waveform Attribute(5:"Valve signal", 6:"NI_LineNames" ("name"), 7:w387) -> (3:w322:digitalwaveform)  [unwired: 1 in, 2 out]
          n208 = case shown="False" "Use Default valve" {
            tunnel: w322 -> [w443 w448]
            tunnel: w321 -> [w442 w446]
            tunnel: [w441 w447] -> w323
            tunnel: w320 -> [_ w445]
            frame False {
              n209 = call-poly <vilib>:"Append Digital Signals.vi"("digital waveform (low bits)"=w442, "digital waveform (high bits)"=w443) -> ("digital waveform out"=w441:digitalwaveform)  [unwired: 8 in, 1 out]
            }
            frame True {
              n210 = call-poly <vilib>:"Append Digital Signals.vi"("digital waveform (low bits)"=w446, "digital waveform (high bits)"=w445) -> ("digital waveform out"=w444:digitalwaveform)  [unwired: 8 in, 1 out]
              n211 = call-poly <vilib>:"Append Digital Signals.vi"("digital waveform (low bits)"=w444, "digital waveform (high bits)"=w448) -> ("digital waveform out"=w447:digitalwaveform)  [unwired: 8 in, 1 out]
            }
          }
          n212 = call-poly <vilib>:"DAQmx Write.vi"("task/channels in"=w423, "auto start"=FALSE, "data"=w323, "error in"=w422) -> ("task out"=w421:refnum<k21>, "error out"=w420:errorcluster)  [unwired: 9 in, 1 out]
          n213 = call <vilib>:"DAQmx Start Task.vi"("task/channels in"=w356, "error in"=w303) -> ("task out"=w304:refnum<k21>, "error out"=w302:errorcluster)  [unwired: 12 in]
          n214 = call <vilib>:"DAQmx Start Task.vi"("task/channels in"=w421, "error in"=w420) -> ("task out"=w425:refnum<k21>, "error out"=w424:errorcluster)  [unwired: 12 in]
          n215 = flat-sequence {
            tunnel: [w596] -> w431
            tunnel: [w595] -> w430
            tunnel: w428 -> [w594]
            tunnel: w427 -> [w597]
            tunnel: [w606] -> w416
            tunnel: w425 -> [w606]
            tunnel: [w605] -> w415
            tunnel: w424 -> [w605]
            tunnel: [w604] -> w368
            tunnel: w304 -> [w603]
            tunnel: w302 -> [w602]
            tunnel: [w603] -> w355
            tunnel: [w602] -> w354
            tunnel: bool[] [FALSE, FALSE, FALSE] ("data") -> [w601]
            tunnel: [w601] -> w352
            tunnel: [w600] -> w350
            tunnel: w351 -> [w600]
            tunnel: [w599] -> w348
            tunnel: w317 -> [w599]
            tunnel: [w598] -> w347
            tunnel: w298 -> [w598]
            frame #0 {
              n216 = Tick Count (ms)() -> (millisecond timer value=w604:u32)
              n217 = call <vilib>:"DAQmx Start Task.vi"("task/channels in"=w597, "error in"=w594) -> ("task out"=w596:refnum<k21>, "error out"=w595:errorcluster)  [unwired: 12 in]
            }
          }
          n218 = call-poly <vilib>:"Digital to Boolean Array.vi"("digital waveform"=w323) -> ()  [unwired: 9 in, 2 out]
          n219 = disable-structure shown="Aktiviert" {
            disable-tunnel: w431 -> [w538 _]
            disable-tunnel: w430 -> [w537 _]
            disable-tunnel: [w536 _] -> w372
            disable-tunnel: [w535 _] -> w373
            disable-tunnel: w416 -> [w534 _]
            disable-tunnel: w415 -> [w533 _]
            disable-tunnel: [w532 _] -> w414
            disable-tunnel: [w531 _] -> w367
            disable-tunnel: w368 -> [w530 _]
            disable-tunnel: w361 -> [w529 _]
            disable-tunnel: w355 -> [w519 _]
            disable-tunnel: w354 -> [w528 _]
            disable-tunnel: w352 -> [w527 _]
            disable-tunnel: w350 -> [w526 _]
            disable-tunnel: [w525 _] -> w349
            disable-tunnel: w348 -> [w524 _]
            disable-tunnel: w347 -> [w523 _]
            disable-tunnel: [w522 _] -> w345
            disable-tunnel: [w521 _] -> w343
            disable-tunnel: [w520 _] -> w310
            frame Enabled {
              n220 = while {
                shift-right: [w574] -> w535
                shift-left: w538 -> [w576]
                shift-right: [w573] -> w536
                shift-left: w537 -> [w575]
                tunnel: w534 -> [w572]
                tunnel: w533 -> [w557]
                tunnel: [w542] -> w532
                tunnel: [w540] -> w531
                tunnel: w530 -> [w567]
                tunnel: w529 -> [w564]
                tunnel: w519 -> [w556]
                tunnel: w528 -> [w554]
                tunnel: [w555] -> w520
                tunnel: [w553] -> w525
                shift-right: [w549] -> _
                shift-left: w527 -> [w552]
                shift-right: [w546] -> w522
                shift-left: w526 -> [w547]
                tunnel: w524 -> [w545]
                tunnel: w523 -> [w544]
                tunnel: [w543] -> w521
                stop <- w568 stop-if-true
                n221 = call-poly <vilib>:"DAQmx Read.vi"("task/channels in"=w556, "error in"=w554) -> ("task out"=w555:refnum<k21>, "data"=w548:u32, "error out"=w553:errorcluster)  [unwired: 11 in]
                "Framecount" <- w548
                n222 = call-poly <vilib>:"DAQmx Read.vi"("task/channels in"=w572, "error in"=w557) -> ("task out"=w558:refnum<k21>, "data"=w549:bool[], "error out"=w541:errorcluster)  [unwired: 11 in]
                n223 = Not Equal?(x=w549, y=w552) -> (x != y?=w551:bool[])
                n224 = Or Array Elements(Boolean array=w551) -> (logical OR=w550:bool)
                n225 = Tick Count (ms)() -> (millisecond timer value=w565:u32)
                n226 = case shown="True" w550 {
                  tunnel: w549 -> [_ w590]
                  tunnel: w548 -> [_ w588]
                  tunnel: w547 -> [w579 w592]
                  tunnel: [w579 w591] -> w546
                  tunnel: w545 -> [_ w582]
                  tunnel: w544 -> [_ w585]
                  tunnel: [errorcluster {"status"=FALSE, "code"=0, "source"=""} ("error out") w581] -> w543
                  frame False {
                  }
                  frame True {
                    w583 = "\t"
                    n227 = Boolean To (0,1)(Boolean=w590) -> (0, 1=w589:i16[])
                    n228 = Number To Decimal String(number=w589) -> (decimal integer string=w586:string[])  [unwired: 1 in]
                    n229 = Number To Decimal String(number=w588) -> (decimal integer string=w587:string)  [unwired: 1 in]
                    n230 = Number To Decimal String(number=w585) -> (decimal integer string=w584:string)  [unwired: 1 in]
                    n231 = Concatenate Strings(w587, w583, w586, w583, w584, w583, w582, "\r\n") -> (w593:string)
                    n232 = Write to Text File(file (use dialog)=w592, text=w593) -> (refnum out=w591:refnum<file>, error out=w581:errorcluster)  [unwired: 2 in, 1 out]
                  }
                }
                n233 = Wait (ms)(milliseconds to wait=u32 1 ("Zu wartende ms")) -> ()  [unwired: 1 out]
                n234 = call <vilib>:"DAQmx Is Task Done.vi"("task/channels in"=w558, "error in"=w541) -> ("task out"=w542:refnum<k21>, "task done?"=w539:bool, "error out"=w540:errorcluster)  [unwired: 11 in]
                n235 = Subtract(x=w565, y=w567) -> (x-y=w560:u32)
                n236 = local read "Stop Boolesch"() -> (w569:bool)
                n237 = call <vilib>:"DAQmx Is Task Done.vi"("task/channels in"=w576, "error in"=w575) -> ("task out"=w574:refnum<k21>, "error out"=w573:errorcluster)  [unwired: 11 in, 1 out]
                n238 = Subtract(x=w565, y=w564) -> (x-y=w562:u32)
                n239 = Divide(x=w560, y=u32 1000 ("x")) -> (x/y=→"Trial elapsed time":dbl)
                n240 = Unbundle By Name(w540) -> ("status"=w570:bool)
                n241 = Divide(x=w562, y=u32 1000 ("x")) -> (x/y=→"Total elapsed time":dbl)
                n242 = Or(x=w570, y=w569) -> (x .or. y?=w577:bool)
                n243 = Or(x=w539, y=w577) -> (x .or. y?=w568:bool)
              }
            }
            frame Disabled {
            }
          }
          n244 = local write "Digitaler output"(w323) -> ()
          n245 = disable-structure shown="Enabled" {
            disable-tunnel: w414 -> [w461 w463]
            disable-tunnel: [w460 w463] -> w371
            disable-tunnel: w367 -> [w459 w462]
            disable-tunnel: [w458 w462] -> w366
            frame Enabled {
              n246 = call <vilib>:"DAQmx Wait Until Done.vi"("task/channels in"=w461, "error in"=w459) -> ("task out"=w460:refnum<k21>, "error out"=w458:errorcluster)  [unwired: 12 in]
            }
            frame Disabled {
            }
          }
          n247 = flat-sequence {
            tunnel: w373 -> [w503]
            tunnel: w372 -> [w492]
            tunnel: w371 -> [w502]
            tunnel: w366 -> [w494]
            tunnel: w349 -> [w497]
            tunnel: w310 -> [w500]
            tunnel: w361 -> [w506]
            frame #0 {
              n248 = call <vilib>:"DAQmx Stop Task.vi"("task/channels in"=w500, "error in"=w497) -> ("task out"=w499:refnum<k21>, "error out"=w498:errorcluster)  [unwired: 12 in]
              n249 = call <vilib>:"DAQmx Stop Task.vi"("task/channels in"=w502, "error in"=w494) -> ("task out"=w495:refnum<k21>, "error out"=w493:errorcluster)  [unwired: 12 in]
              n250 = call <vilib>:"DAQmx Stop Task.vi"("task/channels in"=w503, "error in"=w492) -> ("task out"=w496:refnum<k21>, "error out"=w491:errorcluster)  [unwired: 12 in]
              n251 = call <vilib>:"DAQmx Clear Task.vi"("task in"=w499, "error in"=w498) -> ("error out"=w501:errorcluster)  [unwired: 13 in]
              n252 = call <vilib>:"DAQmx Clear Task.vi"("task in"=w496, "error in"=w491) -> ("error out"=w504:errorcluster)  [unwired: 13 in]
              n253 = call <vilib>:"DAQmx Clear Task.vi"("task in"=w495, "error in"=w493) -> ("error out"=w505:errorcluster)  [unwired: 13 in]
              n254 = Merge Errors(w504, w505, w501) -> ()  [unwired: 1 out]
            }
            frame #1 {
              n255 = Tick Count (ms)() -> (millisecond timer value=w507:u32)
              n256 = for {
                N: "Time between trials" -> [_]
                tunnel: w507 -> [w517]
                tunnel: w506 -> [w512]
                stop <- w510 stop-if-true
                w514 = u32 1000 ("Zu wartende ms")
                n257 = Tick Count (ms)() -> (millisecond timer value=w511:u32)
                n258 = Subtract(x=w511, y=w517) -> (x-y=w518:u32)
                n259 = Subtract(x=w511, y=w512) -> (x-y=w515:u32)
                n260 = local read "Stop Boolesch"() -> (w510:bool)
                n261 = Divide(x=w518, y=w514) -> (x/y=→"Pause elapsed time":dbl)
                n262 = Divide(x=w515, y=w514) -> (x/y=w513:dbl)
                n263 = local write "Total elapsed time"(w513) -> ()
                n264 = Wait (ms)(milliseconds to wait=w514) -> ()  [unwired: 1 out]
              }
              "In between trials" <- TRUE ("In between trials")
            }
          }
          n265 = local read "Stop Boolesch"() -> (w374:bool)
          "Current Valve" <- w365
          "Current list index" <- w370
        }
        n266 = local write "Experiment running"(TRUE ("Experiment running")) -> ()
        n267 = Close File(refnum=w283, error in=w282) -> ()  [unwired: 2 out]
        "State" <- w288
      }
      frame "Stop" {
        n268 = local write "State"(w607) -> ()
        n269 = flat-sequence {
          frame #0 {
            # "Stop-all to zero"
            # "all lines also trigger line"
            n270 = call-poly <vilib>:"DAQmx Write.vi"("task/channels in"="/Dev2/port0/line17:25" ("string"), "data"=bool[] [FALSE, FALSE, FALSE, FALSE, FALSE, FALSE, FALSE, FALSE, FALSE]) -> ("task out"=w615:refnum<k21>, "error out"=w610:errorcluster)  [unwired: 11 in, 1 out]
            n271 = call <vilib>:"DAQmx Start Task.vi"("task/channels in"=w615, "error in"=w610) -> ("task out"=w614:refnum<k21>, "error out"=w612:errorcluster)  [unwired: 12 in]
            n272 = call <vilib>:"DAQmx Wait Until Done.vi"("task/channels in"=w614, "error in"=w612) -> ("task out"=w613:refnum<k21>, "error out"=w611:errorcluster)  [unwired: 12 in]
            n273 = call <vilib>:"DAQmx Clear Task.vi"("task in"=w613, "error in"=w611) -> ()  [unwired: 13 in, 1 out]
          }
          frame #1 {
            w618 = T6."Enabled" ("Deaktiviert")
            n274 = property on="Select experiment" class="TabCtl (strict)"() -> ("Pages"=w621:refnum<vi>[])  [unwired: 2 in, 2 out]
            n275 = property on="Valve order list" class="Arr (strict)"("DisabledEnum"=T6."Enabled" ("Deaktiviert")) -> ()  [unwired: 2 in, 2 out]
            n276 = for {
              tunnel: w621 -> [w622] mode=indexing
              n277 = property class="Page"(reference=w622, "PageEnb"=T7."Page Enabled" ("Aktiv-Status der Seite")) -> ()  [unwired: 1 in, 2 out]
            }
            n278 = property on="Start trial series" class="Bool"("DisabledEnum"=w618) -> ()  [unwired: 2 in, 2 out]
            n279 = property on="Start single trial" class="Bool"("DisabledEnum"=w618) -> ()  [unwired: 2 in, 2 out]
            n280 = property on="Image count filepath" class="Path"("DisabledEnum"=w618) -> ()  [unwired: 2 in, 2 out]
            "Experiment running" <- FALSE ("Experiment running")
          }
        }
        n281 = local read "Stop Boolesch"() -> (w609:bool)
      }
    }
  }
  n282 = while {
    tunnel: w3 -> [w637]
    tunnel: w2 -> [w636]
    shift-right: [w629] -> _
    shift-left: FALSE -> [w634]
    shift-right: [w631] -> _
    shift-left: T1 refnum ("AVI Refnum (duplicate)") -> [w630]
    shift-right: [w627] -> _
    shift-left: refnum<file> refnum ("refnum out") -> [w628]
    stop <- w635 stop-if-true
    n283 = Wait (ms)(milliseconds to wait="Time between frames (ms)") -> ()  [unwired: 1 out]
    n284 = call <vilib>:"IMAQdx Grab2.vi"("Image In"=w636, "Session In"=w637) -> ("Image Out"=w632:T3)  [unwired: 6 in, 3 out]
    "Image" <- w632
    n285 = case shown="False" "Start Recording" {
      tunnel: w634 -> [w642 w656]
      tunnel: w632 -> [_ w663]
      tunnel: [w639 w660] -> w631
      tunnel: w630 -> [w644 w664]
      tunnel: [FALSE w655] -> w629
      tunnel: w628 -> [w643 w662]
      tunnel: [w640 w661] -> w627
      tunnel: "Video path" -> [_ w659]
      tunnel: "Basename" -> [_ w658]
      tunnel: "Save Video as" -> [w641 w657]
      frame False {
        n286 = case shown="False" w642 {
          tunnel: w644 -> [w647 w651]
          tunnel: w643 -> [w646 w648]
          tunnel: w641 -> [_ w652]
          tunnel: [w646 refnum<file> refnum ("refnum out")] -> w640
          tunnel: [w647 T1 refnum ("AVI Refnum (duplicate)")] -> w639
          frame False {
          }
          frame True {
            n287 = case shown="\"Avi\"" w652 {
              tunnel: w651 -> [_ w654]
              tunnel: w648 -> [w653 _]
              frame "Bin", Default {
                n288 = Close File(refnum=w653) -> ()  [unwired: 1 in, 2 out]
              }
              frame "Avi" {
                n289 = call "IMAQ AVI2 Close"("AVI Refnum"=w654) -> ()  [unwired: 10 in, 1 out]
              }
            }
          }
        }
      }
      frame True {
        n290 = case shown="True" w656 {
          tunnel: [w672 w706] -> w660
          tunnel: w664 -> [w670 w707]
          tunnel: w663 -> [w673 w705]
          tunnel: w662 -> [w669 w709]
          tunnel: [w671 w708] -> w661
          tunnel: w659 -> [w668 _]
          tunnel: w658 -> [w667 _]
          tunnel: w657 -> [w666 w704]
          tunnel: w656 -> [_ w703]
          tunnel: [TRUE w703] -> w655
          frame False {
            # "Video recording starts"
            n291 = case shown="\"Avi\"" w666 {
              tunnel: w673 -> [w678 w700]
              tunnel: [w681 w699] -> w672
              tunnel: w668 -> [w684 w697]
              tunnel: w667 -> [w685 w696]
              tunnel: w670 -> [w681 _]
              tunnel: [w679 w695] -> w671
              tunnel: w669 -> [_ w695]
              frame "Bin", Default {
                w675 = FALSE ("prepend array or string size? (T)")
                w676 = T9."little-endian" ("byte order (0:big-endian, network order)")
                n292 = Concatenate Strings(w685, ".bin" ("string")) -> (w692:string)
                n293 = Build Path(base path=w684, name or relative path=w692) -> (appended path=w691:path)
                n294 = Open/Create/Replace File(file path (use dialog)=w691, operation (0:open)=T8."create", access (0:read/write)=enum16{"read/write", "read-only", "write-only"}."write-only") -> (refnum out=w690:refnum<file>, error out=w688:errorcluster)  [unwired: 3 in, 1 out]
                n295 = call "IMAQ GetImageSize"("Image"=w678) -> ("Y Resolution"=w683:i32, "X Resolution"=w682:i32)  [unwired: 3 in, 1 out]
                n296 = Build Array(w682, w683) -> (w689:i32[])
                n297 = Write to Binary File(file (use dialog)=w690, data=w689, error in=w688, 5:w675, 9:w676) -> (refnum out=w680:refnum<file>)  [unwired: 1 in, 2 out]
                n298 = call "IMAQ ImageToArray"("Image"=w678) -> ("Image Pixels (U8)"=w677:u8[][])  [unwired: 3 in, 4 out]
                n299 = Write to Binary File(file (use dialog)=w680, data=w677, 5:w675, 9:w676) -> (refnum out=w679:refnum<file>)  [unwired: 2 in, 2 out]
              }
              frame "Avi" {
                n300 = Concatenate Strings(w696, ".avi" ("string")) -> (w702:string)
                n301 = property on="Avi Codec" class="Ring (strict)"() -> ("RingText.Text"=w693:string)  [unwired: 2 in, 2 out]
                n302 = Build Path(base path=w697, name or relative path=w702) -> (appended path=w698:path)
                n303 = call "IMAQ AVI2 Create"("Codec"=w693, "AVI Path"=w698) -> ("AVI Refnum"=w701:T1)  [unwired: 8 in, 1 out]
                "Experiment Refnum" <- w701
                n304 = call "IMAQ AVI2 Write Frame"("Image"=w700, "AVI Refnum"=w701) -> ("AVI Refnum (duplicate)"=w699:T1)  [unwired: 7 in, 2 out]
              }
            }
          }
          frame True {
            n305 = case shown="\"Bin\", Default" w704 {
              tunnel: w705 -> [w714 w720]
              tunnel: [w711 w719] -> w706
              tunnel: w707 -> [w711 w718]
              tunnel: w709 -> [w713 w717]
              tunnel: [w712 w717] -> w708
              frame "Bin", Default {
                n306 = call "IMAQ ImageToArray"("Image"=w714) -> ("Image Pixels (U8)"=w715:u8[][])  [unwired: 3 in, 4 out]
                n307 = Write to Binary File(file (use dialog)=w713, data=w715, 5:FALSE ("prepend array or string size? (T)"), 9:T9."little-endian" ("byte order (0:big-endian, network order)")) -> (refnum out=w712:refnum<file>)  [unwired: 2 in, 2 out]
              }
              frame "Avi" {
                n308 = call "IMAQ AVI2 Write Frame"("Image"=w720, "AVI Refnum"=w718) -> ("AVI Refnum (duplicate)"=w719:T1)  [unwired: 7 in, 2 out]
              }
            }
          }
        }
      }
    }
    n309 = local read "Stop Boolesch"() -> (w635:bool)
  }
  n310 = while {
    tunnel: w16 -> [w722]
    stop <- w721 stop-if-true
    n311 = event shown="[3] \"Load exp. ini\": Value Change" {
      selector: _ -> [_ _ _ _ _]
      dyn-events: _ -> [_ _ _ _ _]
      timeout: _ -> [_ _ _ _ _]
      tunnel: w722 -> [_ w723 w732 _ w787]
      event Timeout {
        n312 = event-data() -> ()  [unwired: 1 in, 3 out]
      }
      event "Start single trial": Value Change {
        n313 = event-data() -> ()  [unwired: 1 in, 6 out]
        n314 = case shown="True" "Start single trial" {
          tunnel: w723 -> [_ w731]
          frame False {
          }
          frame True {
            n315 = property on="Start single trial" class="Bool"("DisabledEnum"=T6."Disabled and Grayed Out" ("Deaktiviert")) -> ()  [unwired: 2 in, 2 out]
            n316 = Enqueue Element(queue=w731, element=StatesEnum."Start Trial" ("Enum")) -> ()  [unwired: 2 in, 3 out]
            n317 = property on="Select experiment" class="TabCtl (strict)"() -> ("Pages"=w727:refnum<vi>[])  [unwired: 2 in, 2 out]
            n318 = Index Array(array=w727, index=1 ("Index")) -> (element=w728:refnum<vi>)
            n319 = property class="Page"(reference=w728, "PageEnb"=T7."Page Disabled & Grayed" ("Aktiv-Status der Seite")) -> ()  [unwired: 1 in, 2 out]
          }
        }
      }
      event "Stopp": Value Change {
        n320 = event-data() -> ()  [unwired: 1 in, 6 out]
        n321 = case shown="True" "Stopp" {
          tunnel: w732 -> [_ w736]
          frame False {
          }
          frame True {
            n322 = Enqueue Element(queue=w736, element=StatesEnum."Stop" ("Enum")) -> ()  [unwired: 2 in, 3 out]
            "Stop Boolesch" <- TRUE ("Stop Boolesch")
          }
        }
      }
      event "Load exp. ini": Value Change {
        n323 = event-data() -> ()  [unwired: 1 in, 6 out]
        n324 = case shown="True" "Load exp. ini" {
          frame False {
          }
          frame True {
            n325 = call "File Dialog"("prompt"="Please select an experiment ini file", "pattern (all files)"="*.ini") -> ("selected path"=w738:path, "cancelled"=w739:bool)  [unwired: 10 in, 2 out]
            n326 = case shown="False" w739 {
              tunnel: w738 -> [w780 _]
              frame False {
                w752 = "Odor System" ("section")
                n327 = call <vilib>:"Open Config Data.vi"("configuration file path"=w780) -> ("error out"=w778:errorcluster, "refnum"=w779:T10)  [unwired: 8 in, 1 out]
                n328 = call-poly <vilib>:"Read Key.vi"("section"=w752, "error in (no error)"=w778, "key"="Value delay", "refnum"=w779) -> ("error out"=w774:errorcluster, "value"=w776:dbl, "refnum out"=w775:T10)  [unwired: 4 in, 1 out]
                n329 = local write "Valve delay"(w776) -> ()
                n330 = call-poly <vilib>:"Read Key.vi"("section"=w752, "error in (no error)"=w774, "key"="Valve opening time", "refnum"=w775) -> ("error out"=w770:errorcluster, "value"=w772:dbl, "refnum out"=w771:T10)  [unwired: 4 in, 1 out]
                n331 = local write "Valve opening time"(w772) -> ()
                n332 = call-poly <vilib>:"Read Key.vi"("section"=w752, "error in (no error)"=w770, "key"="Total trial time", "refnum"=w771) -> ("error out"=w767:errorcluster, "value"=w768:dbl, "refnum out"=w766:T10)  [unwired: 4 in, 1 out]
                n333 = local write "Total trial time"(w768) -> ()
                n334 = call-poly <vilib>:"Read Key.vi"("section"=w752, "error in (no error)"=w767, "key"="Time between trials", "refnum"=w766) -> ("error out"=w763:errorcluster, "value"=w762:i32, "refnum out"=w764:T10)  [unwired: 4 in, 1 out]
                n335 = local write "Time between trials"(w762) -> ()
                n336 = call-poly <vilib>:"Read Key.vi"("section"=w752, "error in (no error)"=w763, "key"="Use Default valve", "refnum"=w764) -> ("error out"=w758:errorcluster, "value"=w760:bool, "refnum out"=w759:T10)  [unwired: 4 in, 1 out]
                n337 = local write "Use Default valve"(w760) -> ()
                n338 = call-poly <vilib>:"Read Key.vi"("section"=w752, "error in (no error)"=w758, "key"="Selected default valve ", "refnum"=w759) -> ("error out"=w754:errorcluster, "value"=w756:i32, "refnum out"=w755:T10)  [unwired: 4 in, 1 out]
                n339 = local write "Selected default valve"(w756) -> ()
                n340 = call-poly <vilib>:"Read Key.vi"("section"=w752, "error in (no error)"=w754, "key"="Valve order list", "refnum"=w755) -> ("error out"=w747:errorcluster, "value"=w751:string, "refnum out"=w748:T10)  [unwired: 4 in, 1 out]
                n341 = Spreadsheet String To Array(delimiter (Tab)=";", format string="%d", spreadsheet string=w751, array type (2D Dbl)=i8[] [] ("Valve order list")) -> (array=w749:i8[])
                n342 = local write "Valve order list"(w749) -> ()
                n343 = call <vilib>:"Close Config Data.vi"("error in (no error)"=w747, "refnum"=w748) -> ("error out"=w745:errorcluster, "file path"=w744:path)  [unwired: 8 in]
                n344 = Unbundle By Name(w745) -> ("status"=w746:bool)
                n345 = case shown="True" w746 {
                  tunnel: w745 -> [_ w785]
                  tunnel: w744 -> [w782 _]
                  frame False {
                    n346 = Strip Path(path=w782) -> (name=→"Loaded experiment":string)  [unwired: 1 out]
                  }
                  frame True {
                    w784 = T11 3 items=["no dialog", "OK message", "continue or stop message", "OK message + warnings", "continue/stop + warnings"] ("type of dialog (OK msg:1)")
                    n347 = call <vilib>:"Simple Error Handler.vi"("error source (\" \")"="Error loading experiment ini file" ("error source (\" \")"), "type of dialog (OK msg:1)"=w784, "error in (no error)"=w785) -> ()  [unwired: 2 in, 5 out]
                  }
                }
              }
              frame True {
              }
            }
          }
        }
      }
      event "Start trial series": Value Change {
        n348 = event-data() -> ()  [unwired: 1 in, 6 out]
        n349 = case shown="True" "Start trial series" {
          tunnel: w787 -> [_ w794]
          frame False {
          }
          frame True {
            n350 = property on="Start trial series" class="Bool"("DisabledEnum"=T6."Disabled and Grayed Out" ("Deaktiviert")) -> ()  [unwired: 2 in, 2 out]
            n351 = Enqueue Element(queue=w794, element=StatesEnum."Start trial series" ("Enum")) -> ()  [unwired: 2 in, 3 out]
            n352 = property on="Select experiment" class="TabCtl (strict)"() -> ("Pages"=w790:refnum<vi>[])  [unwired: 2 in, 2 out]
            n353 = Index Array(array=w790, index=0 ("Index")) -> (element=w791:refnum<vi>)
            n354 = property class="Page"(reference=w791, "PageEnb"=T7."Page Disabled & Grayed" ("Aktiv-Status der Seite")) -> ()  [unwired: 1 in, 2 out]
          }
        }
      }
    }
    n355 = local read "Stop Boolesch"() -> (w721:bool)
  }
  n356 = Release Queue(queue=w15) -> ()  [unwired: 2 in, 3 out]
